vi "Parse Downlink.vi"(7 "CP_DATA IN":u8[](array[numeric]), 8 "error in (no error)":errorcluster, 9 "Parameters":string, 10 "EXID":u32 step=1 format="%06x", 11 "Command":T1) -> (0 "error out":errorcluster, 2 "Downlink":u8[][](array[numeric]) format="%02x")   [LabVIEW 2009]
uses:
  <vilib>/Utility/miscctls.llb/LVDateTimeRec.ctl
  Command List.ctl
  Typedef Command List.ctl
panel:
  in  "Command":T2 items=["Get xPG Status", "xPG Stimulation", "Select Program", "Increment Program Amplitude", "Decrement Program Amplitude", "Get PoP Constants", "Get PPC Constants", "Get Program Names", "Set Pulse Amplitude", "Increment Pulse Amplitude", "Decrement Pulse Amplitude", "Get Pulse Widths", "Set Pulse Widths", "Increment Pulse Width", "Decrement Pulse Width", "Get Program Frequency", "Set Program Frequency", "Increment Program Frequency", "Decrement Program Frequency", "reserved", "Charging Control", "Get xPG Identity", "Set xPG Identity", "Restore Program Defaults", "Get Program Definition", "Set Program Definition", "Get Program Constants", "Set Program Constants", "Get Configurable Device Parameters", "Set Configurable Device Parameters", "Get Pulse Constants", "Set Pulse Constants", "Get Lead Limits", "Set Lead Limits", "Get Channel Calibrations", "Set Channel Calibrations", "reserved", "reserved", "reserved", "reserved", "reserved", "reserved", "Get Stim Asic HV Calibrations", "Set Stim Asic HV Calibrations", "reserved", "reserved", "Get CP Data", "Set CP Data", "Clear Log", "Read Log", "Append Log", "Get Patient Program Runtime", "Set Patient Program Runtimec", "Impedance Measurement", "Enter Storage Mode", "Echo Short", "Echo Long", "Get General Calibration", "Set General Calibration", "Get Trim List", "Set Trim List", "Get Counter", "Set Counter", "Get Test Stimulation", "Set Test Stimulation", "Get Titration Stimulation", "Set Titration Stimulation", "Get Ramp Time", "Set Ramp Time", "Get VBAT", "Set Software Description Block", "Write Memory", "Read Memory", "Reset xPG", "Erase Flash Block", "Write Vectors", "Read Vectors", "Diagnostic Data", "Set Background Impedance", "Get Background Impedence ", "Undefined"]
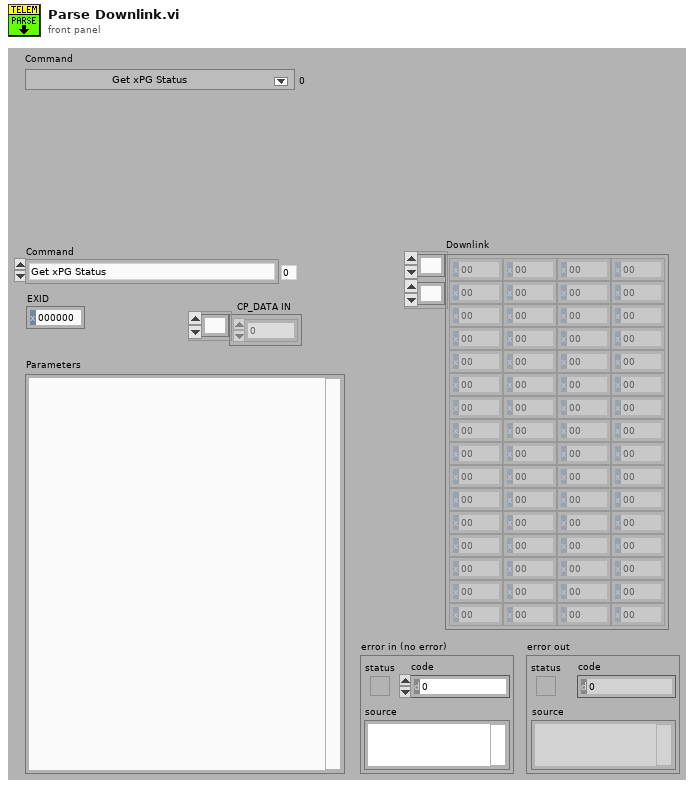
[diagram p1: front panel]
types:
  T1 = typedef "Typedef Command List.ctl" = enum16{"Get xPG Status", "xPG Stimulation", "Select Program", "Increment Program Amplitude", "Decrement Program Amplitude", "Get PoP Constants", "Get PPC Constants", "Get Program Names", "Set Pulse Amplitude", "Increment Pulse Amplitude", "Decrement Pulse Amplitude", "Get Pulse Widths", "Set Pulse Widths", "Increment Pulse Width", "Decrement Pulse Width", "Get Program Frequency", "Set Program Frequency", "Increment Program Frequency", "Decrement Program Frequency", "<reserved 1>", "Charging Control", "Get xPG Identity", "Set xPG Identity", "Restore Program Defaults", "Get Program Definition", "Set Program Definition", "Get Program Constants", "Set Program Constants", "Get Configurable Device Parameters", "Set Configurable Device Parameters", "Get Pulse Constants", "Set Pulse Constants", "Get Lead Limits", "Set Lead Limits", "Get Channel Calibrations", "Set Channel Calibrations", "<reserved 2>", "<reserved 3>", "<reserved 4>", "<reserved 5>", "<reserved 6>", "<reserved 7>", "Get Stim Asic HV Calibrations", "Set Stim Asic HV Calibrations", "<reserved 8>", "<reserved 9>", "Get CP Data", "Set CP Data", "Clear Log", "Read Log", "Append Log", "Get Patient Program Runtime", "Set Patient Program Runtime", "Impedance Measurement", "Enter Storage Mode", "Echo Short", "Echo Long", "Get General Calibration", "Set General Calibration", "Get Trim List", "Set Trim List", "Get Counter", "Set Counter", "Get Test Stimulation", "Set Test Stimulation", "Get Titration Stimulation", "Set Titration Stimulation", "Get Ramp Time", "Set Ramp Time", "Get VBAT", "Set Software Description Block", "Get Software Description Block", "Write Memory", "Read Memory", "Reset xPG", "Erase Flash Block", "Write Vectors", "Read Vectors", "Diagnostic Data", "Set Background Impedance", "Get Background Impedence ", "Undefined"}
  T2 = typedef "Command List.ctl" = u16
  T3 = enum16{"U8", "U16", "U32", "U64", "I8", "I16", "I32", "I64"}
  T4 = typedef "LVDateTimeRec.ctl" = cluster{"fractional second":dbl, "second":i32, "minute":i32, "hour":i32, "day of month":i32, "month":i32, "year":i32, "day of week":i32, "day of year":i32, "DST":i32}
  T5 = cluster{"CP_DATA IN[0]":u8, "CP_DATA IN[1]":u8, "CP_DATA IN[2]":u8, "CP_DATA IN[3]":u8, "CP_DATA IN[4]":u8, "CP_DATA IN[5]":u8, "CP_DATA IN[6]":u8, "CP_DATA IN[7]":u8, "CP_DATA IN[8]":u8, "CP_DATA IN[9]":u8, "CP_DATA IN[10]":u8, "CP_DATA IN[11]":u8, "CP_DATA IN[12]":u8, "CP_DATA IN[13]":u8, "CP_DATA IN[14]":u8, "CP_DATA IN[15]":u8, "CP_DATA IN[16]":u8, "CP_DATA IN[17]":u8, "CP_DATA IN[18]":u8, "CP_DATA IN[19]":u8, "CP_DATA IN[20]":u8, "CP_DATA IN[21]":u8, "CP_DATA IN[22]":u8, "CP_DATA IN[23]":u8, "CP_DATA IN[24]":u8, "CP_DATA IN[25]":u8, "CP_DATA IN[26]":u8, "CP_DATA IN[27]":u8, "CP_DATA IN[28]":u8, "CP_DATA IN[29]":u8, "CP_DATA IN[30]":u8, "CP_DATA IN[31]":u8, "CP_DATA IN[32]":u8, "CP_DATA IN[33]":u8, "CP_DATA IN[34]":u8, "CP_DATA IN[35]":u8, "CP_DATA IN[36]":u8, "CP_DATA IN[37]":u8, "CP_DATA IN[38]":u8, "CP_DATA IN[39]":u8, "CP_DATA IN[40]":u8, "CP_DATA IN[41]":u8, "CP_DATA IN[42]":u8, "CP_DATA IN[43]":u8, "CP_DATA IN[44]":u8, "CP_DATA IN[45]":u8, "CP_DATA IN[46]":u8, "CP_DATA IN[47]":u8, "CP_DATA IN[48]":u8, "CP_DATA IN[49]":u8, "CP_DATA IN[50]":u8, "CP_DATA IN[51]":u8, "CP_DATA IN[52]":u8, "CP_DATA IN[53]":u8, "CP_DATA IN[54]":u8, "CP_DATA IN[55]":u8, "CP_DATA IN[56]":u8, "CP_DATA IN[57]":u8, "CP_DATA IN[58]":u8, "CP_DATA IN[59]":u8, "CP_DATA IN[60]":u8, "CP_DATA IN[61]":u8, "CP_DATA IN[62]":u8, "CP_DATA IN[63]":u8, "CP_DATA IN[64]":u8, "CP_DATA IN[65]":u8, "CP_DATA IN[66]":u8, "CP_DATA IN[67]":u8, "CP_DATA IN[68]":u8, "CP_DATA IN[69]":u8, "CP_DATA IN[70]":u8, "CP_DATA IN[71]":u8, "CP_DATA IN[72]":u8, "CP_DATA IN[73]":u8, "CP_DATA IN[74]":u8, "CP_DATA IN[75]":u8, "CP_DATA IN[76]":u8, "CP_DATA IN[77]":u8, "CP_DATA IN[78]":u8, "CP_DATA IN[79]":u8, "CP_DATA IN[80]":u8, "CP_DATA IN[81]":u8, "CP_DATA IN[82]":u8, "CP_DATA IN[83]":u8, "CP_DATA IN[84]":u8, "CP_DATA IN[85]":u8, "CP_DATA IN[86]":u8, "CP_DATA IN[87]":u8, "CP_DATA IN[88]":u8, "CP_DATA IN[89]":u8, "CP_DATA IN[90]":u8, "CP_DATA IN[91]":u8, "CP_DATA IN[92]":u8, "CP_DATA IN[93]":u8, "CP_DATA IN[94]":u8, "CP_DATA IN[95]":u8, "CP_DATA IN[96]":u8, "CP_DATA IN[97]":u8, "CP_DATA IN[98]":u8, "CP_DATA IN[99]":u8, "CP_DATA IN[100]":u8, "CP_DATA IN[101]":u8, "CP_DATA IN[102]":u8, "CP_DATA IN[103]":u8, "CP_DATA IN[104]":u8, "CP_DATA IN[105]":u8, "CP_DATA IN[106]":u8, "CP_DATA IN[107]":u8, "CP_DATA IN[108]":u8, "CP_DATA IN[109]":u8, "CP_DATA IN[110]":u8, "CP_DATA IN[111]":u8, "CP_DATA IN[112]":u8, "CP_DATA IN[113]":u8, "CP_DATA IN[114]":u8, "CP_DATA IN[115]":u8, "CP_DATA IN[116]":u8, "CP_DATA IN[117]":u8, "CP_DATA IN[118]":u8, "CP_DATA IN[119]":u8, "CP_DATA IN[120]":u8, "CP_DATA IN[121]":u8, "CP_DATA IN[122]":u8, "CP_DATA IN[123]":u8, "CP_DATA IN[124]":u8, "CP_DATA IN[125]":u8, "CP_DATA IN[126]":u8, "CP_DATA IN[127]":u8, "CP_DATA IN[128]":u8, "CP_DATA IN[129]":u8, "CP_DATA IN[130]":u8, "CP_DATA IN[131]":u8, "CP_DATA IN[132]":u8, "CP_DATA IN[133]":u8, "CP_DATA IN[134]":u8, "CP_DATA IN[135]":u8, "CP_DATA IN[136]":u8, "CP_DATA IN[137]":u8, "CP_DATA IN[138]":u8, "CP_DATA IN[139]":u8, "CP_DATA IN[140]":u8, "CP_DATA IN[141]":u8, "CP_DATA IN[142]":u8, "CP_DATA IN[143]":u8, "CP_DATA IN[144]":u8, "CP_DATA IN[145]":u8, "CP_DATA IN[146]":u8, "CP_DATA IN[147]":u8, "CP_DATA IN[148]":u8, "CP_DATA IN[149]":u8, "CP_DATA IN[150]":u8, "CP_DATA IN[151]":u8, "CP_DATA IN[152]":u8, "CP_DATA IN[153]":u8, "CP_DATA IN[154]":u8, "CP_DATA IN[155]":u8, "CP_DATA IN[156]":u8, "CP_DATA IN[157]":u8, "CP_DATA IN[158]":u8, "CP_DATA IN[159]":u8, "CP_DATA IN[160]":u8, "CP_DATA IN[161]":u8, "CP_DATA IN[162]":u8, "CP_DATA IN[163]":u8, "CP_DATA IN[164]":u8, "CP_DATA IN[165]":u8, "CP_DATA IN[166]":u8, "CP_DATA IN[167]":u8, "CP_DATA IN[168]":u8, "CP_DATA IN[169]":u8, "CP_DATA IN[170]":u8, "CP_DATA IN[171]":u8, "CP_DATA IN[172]":u8, "CP_DATA IN[173]":u8, "CP_DATA IN[174]":u8, "CP_DATA IN[175]":u8, "CP_DATA IN[176]":u8, "CP_DATA IN[177]":u8, "CP_DATA IN[178]":u8, "CP_DATA IN[179]":u8, "CP_DATA IN[180]":u8, "CP_DATA IN[181]":u8, "CP_DATA IN[182]":u8, "CP_DATA IN[183]":u8, "CP_DATA IN[184]":u8, "CP_DATA IN[185]":u8, "CP_DATA IN[186]":u8, "CP_DATA IN[187]":u8, "CP_DATA IN[188]":u8, "CP_DATA IN[189]":u8, "CP_DATA IN[190]":u8, "CP_DATA IN[191]":u8, "CP_DATA IN[192]":u8, "CP_DATA IN[193]":u8, "CP_DATA IN[194]":u8, "CP_DATA IN[195]":u8, "CP_DATA IN[196]":u8, "CP_DATA IN[197]":u8, "CP_DATA IN[198]":u8, "CP_DATA IN[199]":u8, "CP_DATA IN[200]":u8, "CP_DATA IN[201]":u8, "CP_DATA IN[202]":u8, "CP_DATA IN[203]":u8, "CP_DATA IN[204]":u8, "CP_DATA IN[205]":u8, "CP_DATA IN[206]":u8, "CP_DATA IN[207]":u8, "CP_DATA IN[208]":u8, "CP_DATA IN[209]":u8, "CP_DATA IN[210]":u8, "CP_DATA IN[211]":u8, "CP_DATA IN[212]":u8, "CP_DATA IN[213]":u8, "CP_DATA IN[214]":u8, "CP_DATA IN[215]":u8, "CP_DATA IN[216]":u8, "CP_DATA IN[217]":u8, "CP_DATA IN[218]":u8, "CP_DATA IN[219]":u8, "CP_DATA IN[220]":u8, "CP_DATA IN[221]":u8, "CP_DATA IN[222]":u8, "CP_DATA IN[223]":u8, "CP_DATA IN[224]":u8, "CP_DATA IN[225]":u8, "CP_DATA IN[226]":u8, "CP_DATA IN[227]":u8, "CP_DATA IN[228]":u8, "CP_DATA IN[229]":u8, "CP_DATA IN[230]":u8, "CP_DATA IN[231]":u8, "CP_DATA IN[232]":u8, "CP_DATA IN[233]":u8, "CP_DATA IN[234]":u8, "CP_DATA IN[235]":u8, "CP_DATA IN[236]":u8, "CP_DATA IN[237]":u8, "CP_DATA IN[238]":u8, "CP_DATA IN[239]":u8, "CP_DATA IN[240]":u8, "CP_DATA IN[241]":u8, "CP_DATA IN[242]":u8, "CP_DATA IN[243]":u8, "CP_DATA IN[244]":u8, "CP_DATA IN[245]":u8, "CP_DATA IN[246]":u8, "CP_DATA IN[247]":u8, "CP_DATA IN[248]":u8, "CP_DATA IN[249]":u8, "CP_DATA IN[250]":u8, "CP_DATA IN[251]":u8, "CP_DATA IN[252]":u8, "CP_DATA IN[253]":u8, "CP_DATA IN[254]":u8, "CP_DATA IN[255]":u8}
  T6 = cluster{"DATA[0]":u8, "DATA[1]":u8, "DATA[2]":u8, "DATA[3]":u8, "DATA[4]":u8, "DATA[5]":u8, "DATA[6]":u8, "DATA[7]":u8, "DATA[8]":u8, "DATA[9]":u8, "DATA[10]":u8, "DATA[11]":u8, "DATA[12]":u8, "DATA[13]":u8, "DATA[14]":u8}
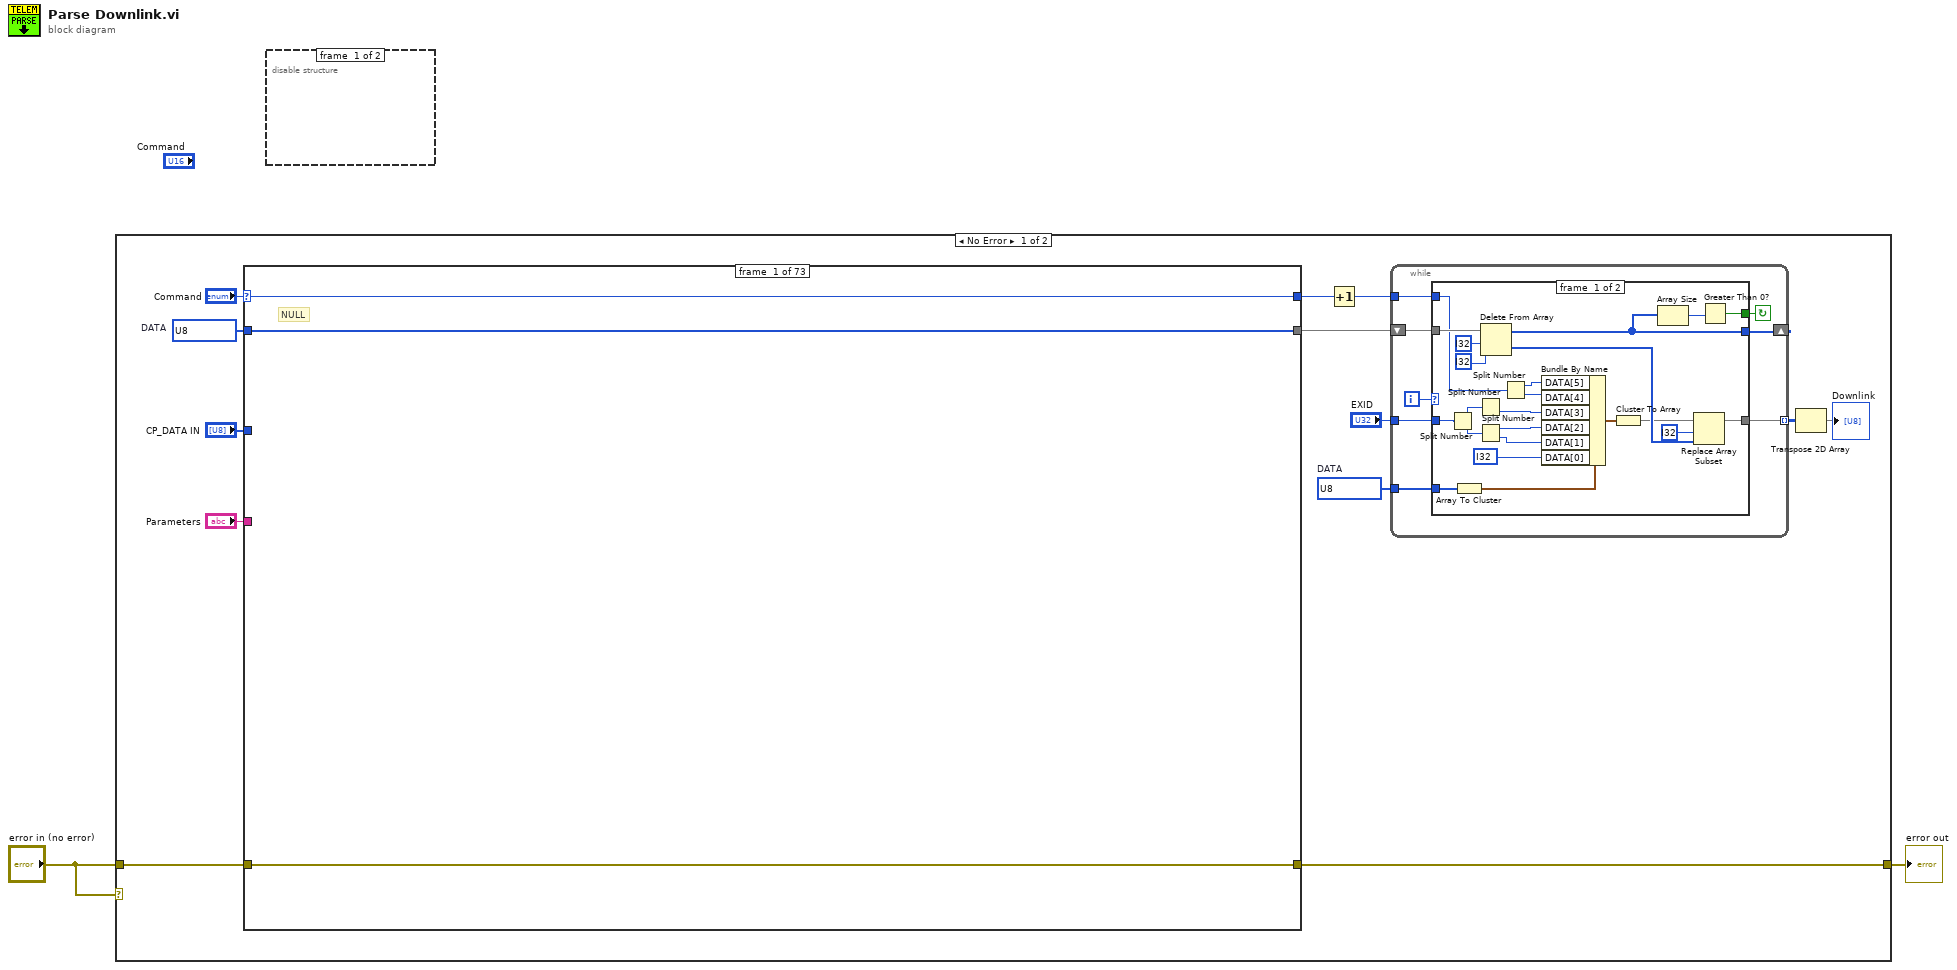
[diagram p0: block diagram]
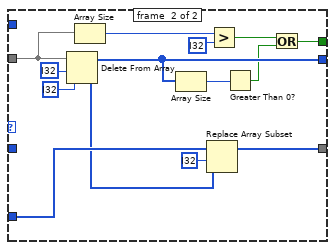
[diagram p3: hidden frame]
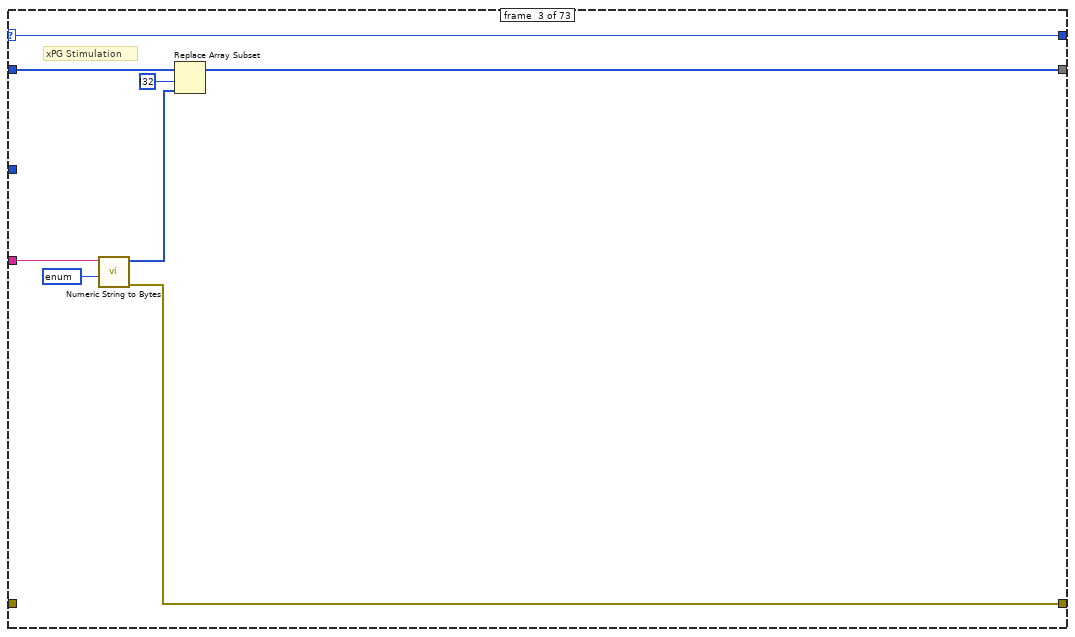
[diagram p5: hidden frame]
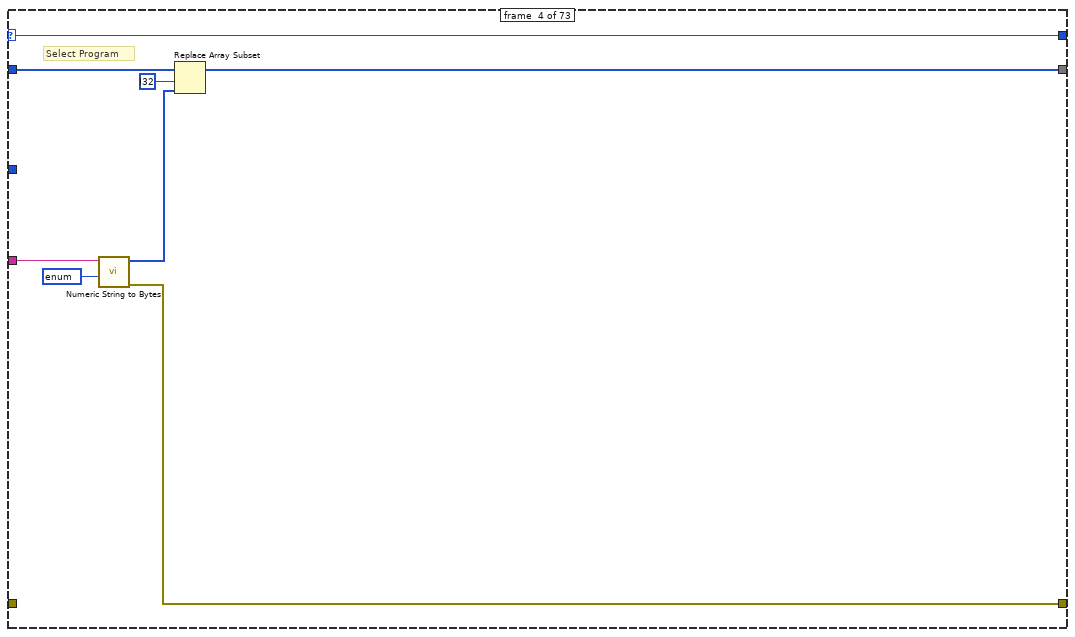
[diagram p6: hidden frame]
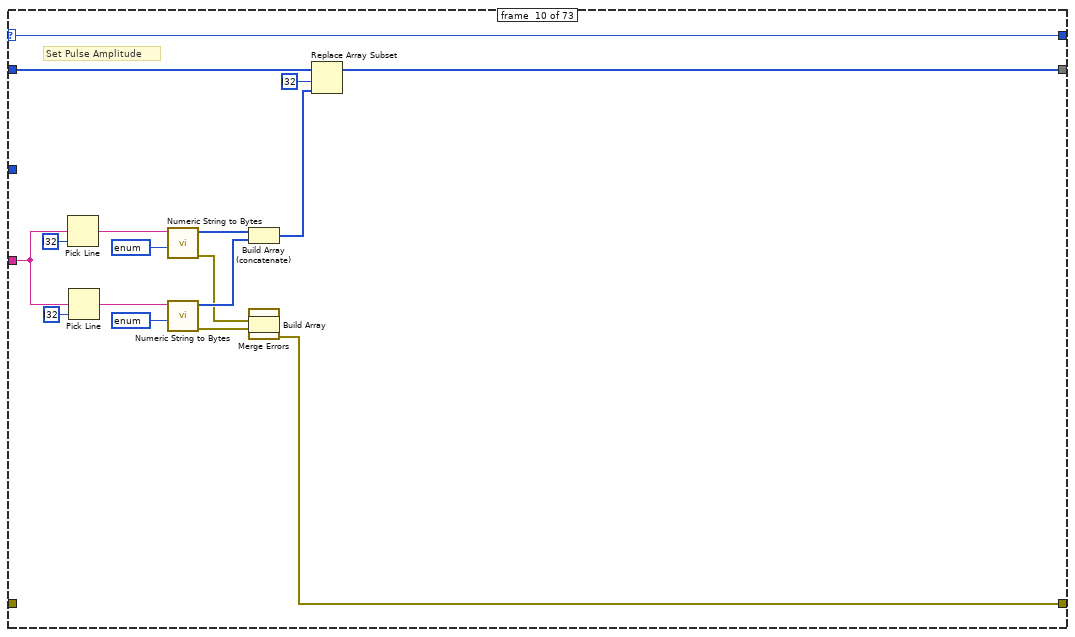
[diagram p12: hidden frame]
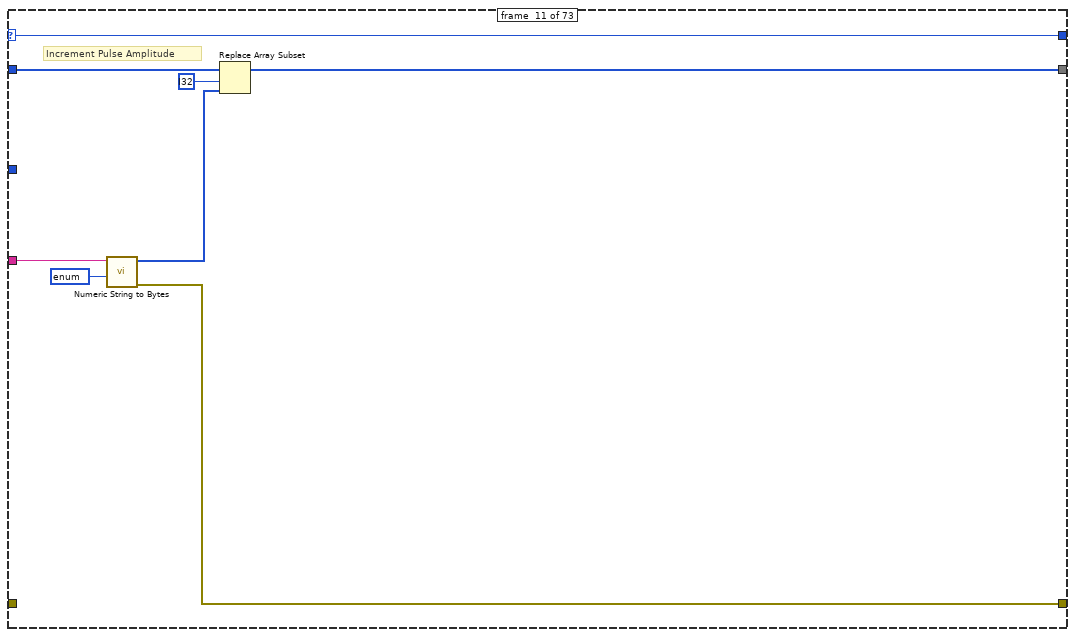
[diagram p13: hidden frame]
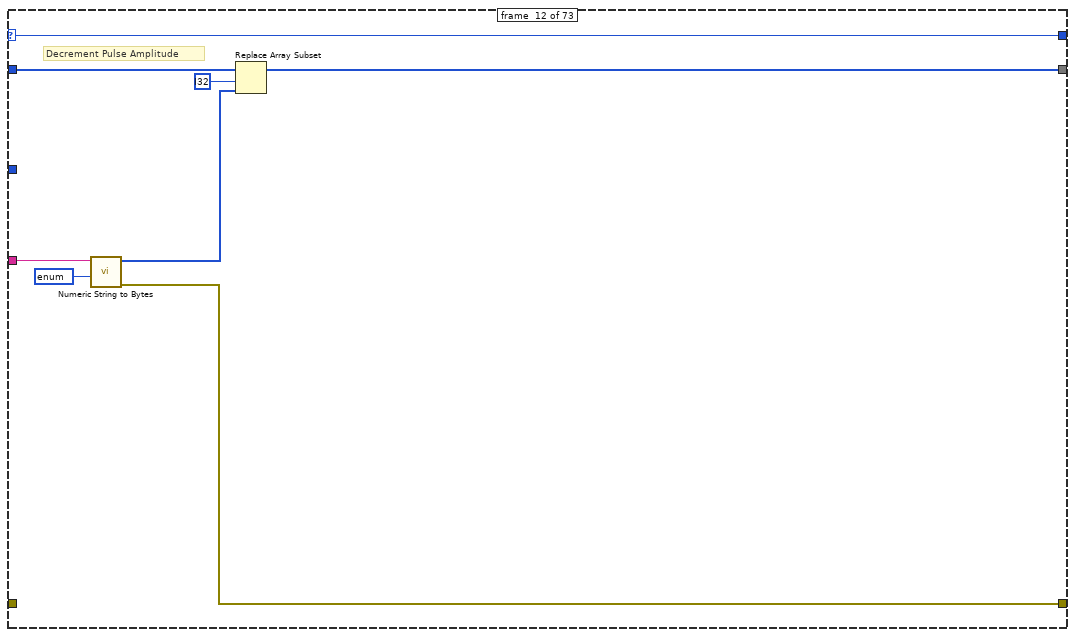
[diagram p14: hidden frame]
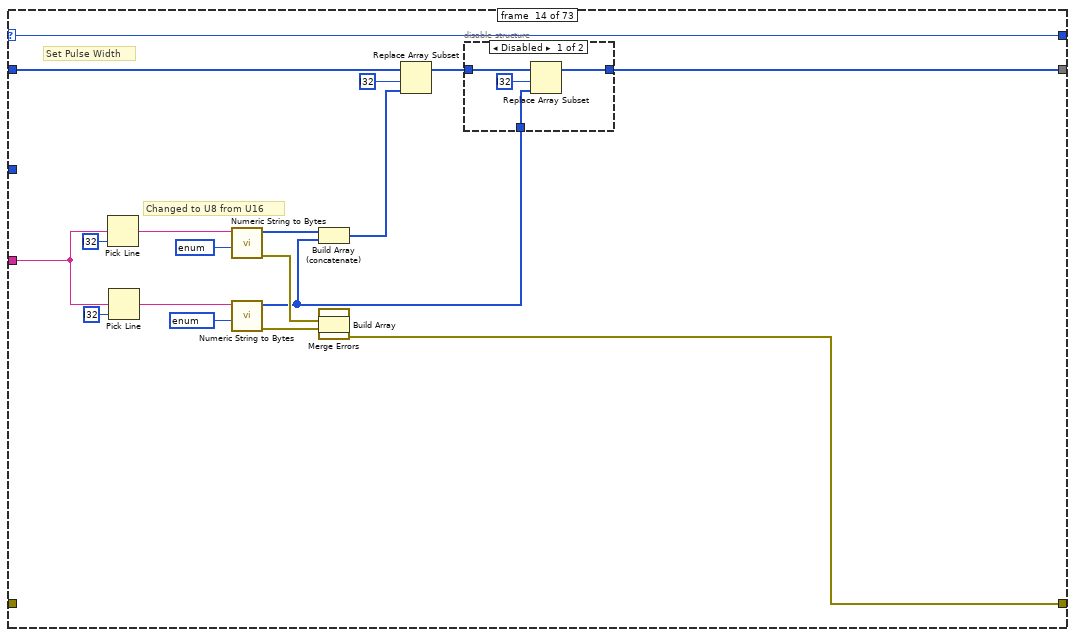
[diagram p16: hidden frame]
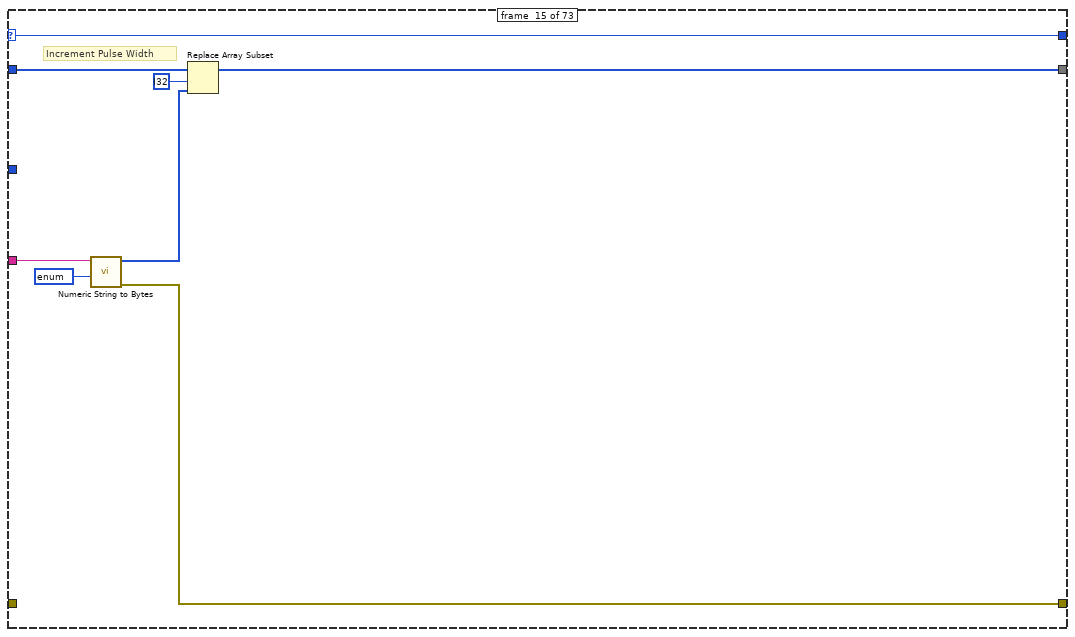
[diagram p18: hidden frame]
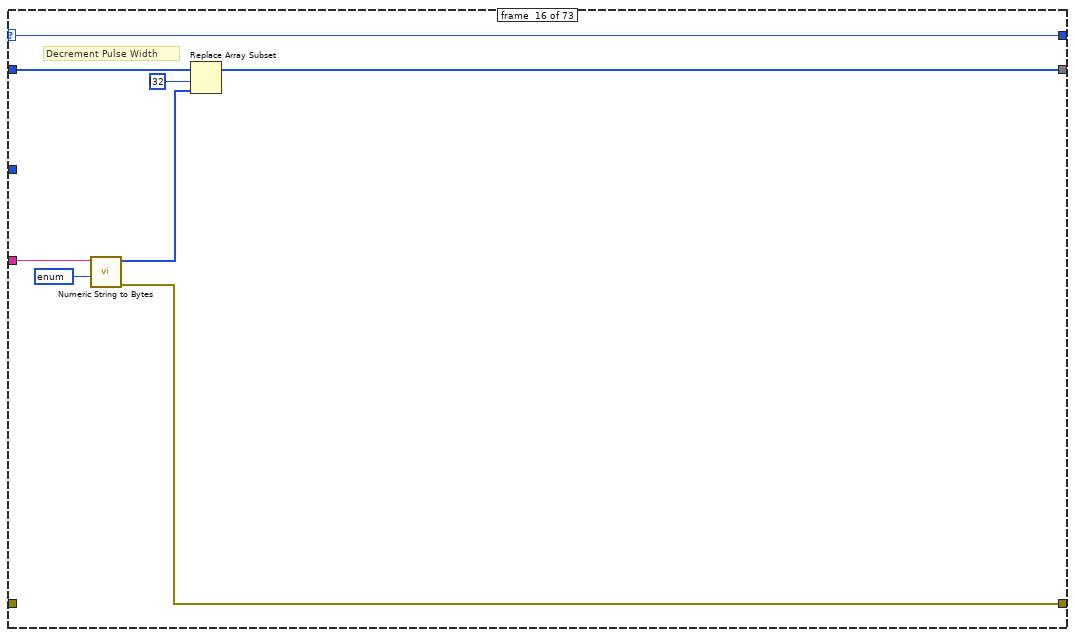
[diagram p19: hidden frame]
diagram:
  n1 = case shown="No Error" "error in (no error)" {
    tunnel: "error in (no error)" -> [w8 w1212]
    tunnel: [w7 w1212] -> w2
    frame #0 {
      w9 = u8[] ?  # DATA
      w10 = u8[] ?  # DATA
      n2 = case shown="\"Set Program Definition\"" "Command" {
        selector: "Command" -> [w63 w66 w74 w82 w85 w88 w91 w94 w97 w115 w123 w131 w134 w153 w166 w174 w177 w185 w188 w191 w194 w197 w224 w240 w248 w255 w395 w410 w423 w498 w516 w536 w547 w555 w566 w574 w585 w593 w609 w622 w630 w649 w688 w696 w715 w769 w772 w778 w784 w787 w794 w896 w918 w943 w962 w965 w989 w1046 w1066 w1099 w1107 w1110 w1113 w1116 w1135 w1153 w1156 w1159 w1162 w1165 w1183 w1208 w1211]
        tunnel: "Parameters" -> [_ _ w72 w80 _ _ _ _ _ w114 w121 w129 _ w141 w164 w172 _ w183 _ _ _ _ w222 w238 w246 w250 _ w398 _ w428 _ w523 _ w552 _ w571 _ w590 w607 w617 w628 w632 w653 w694 w698 w722 _ _ _ _ w790 w891 w906 w941 w945 _ w971 _ w1057 _ w1104 _ _ _ w1124 w1148 _ _ _ _ w1179 w1191 _]
        tunnel: [w63 w66 w74 w82 w85 w88 w91 w94 w97 w115 w123 w131 w134 w153 w166 w174 w177 w185 w188 w191 w194 w197 w224 w240 w248 w255 w395 w410 w423 w498 w516 w536 w547 w555 w566 w574 w585 w593 w609 w622 w630 w649 w688 w696 w715 w769 w772 w778 w784 w787 w794 w896 w918 w943 w962 w965 w989 w1046 w1066 w1099 w1107 w1110 w1113 w1116 w1135 w1153 w1156 w1159 w1162 w1165 w1183 w1208 w1211] -> w15
        tunnel: [w62 w65 w70 w78 w84 w87 w90 w93 w96 w107 w119 w127 w133 w139 w162 w170 w176 w181 w187 w190 w193 w196 w209 w236 w244 w251 w394 w408 w422 w495 w515 w533 w546 w550 w565 w569 w584 w588 w605 w616 w626 w647 w686 w692 w713 w767 w771 w774 w780 w786 w791 w889 w913 w939 w960 w963 w967 w1044 w1052 w1097 w1101 w1108 w1111 w1114 w1123 w1137 w1154 w1157 w1160 w1163 w1167 w1199 w1210] -> w13
        tunnel: w9 -> [w62 w65 w73 w81 w84 w87 w90 w93 w96 w106 w122 w130 w133 w146 w165 w173 w176 w184 w187 w190 w193 w196 w210 w239 w247 _ w394 _ w422 _ w515 _ w546 _ w565 _ w584 _ w608 _ w629 w648 w687 w695 w714 w768 w771 _ _ w786 _ w892 _ w942 w961 w963 _ w1044 _ w1097 w1103 w1108 w1111 w1114 _ w1138 w1154 w1157 w1160 w1163 w1170 _ w1210]
        tunnel: w8 -> [w61 w64 _ _ w83 w86 w89 w92 w95 _ _ _ w132 _ _ _ w175 _ w186 w189 w192 w195 _ _ _ w253 w393 _ w421 _ w514 _ w545 _ w564 _ w583 _ _ _ _ _ _ _ _ _ w770 w773 w779 w785 _ _ _ _ _ w964 _ w1045 _ w1098 _ w1109 w1112 w1115 _ _ w1155 w1158 w1161 w1164 _ _ w1209]
        tunnel: [w61 w64 w71 w79 w83 w86 w89 w92 w95 w99 w120 w128 w132 w142 w163 w171 w175 w182 w186 w189 w192 w195 w199 w237 w245 w252 w393 w401 w421 w496 w514 w532 w545 w553 w564 w572 w583 w591 w606 w621 w627 w633 w672 w693 w699 w753 w770 w773 w779 w785 w792 w890 w917 w940 w946 w964 w969 w1045 w1048 w1098 w1100 w1109 w1112 w1115 w1122 w1139 w1155 w1158 w1161 w1164 w1171 w1185 w1209] -> w7
        tunnel: "CP_DATA IN" -> [_ _ _ _ _ _ _ _ _ _ _ _ _ _ _ _ _ _ _ _ _ _ _ _ _ _ _ _ _ _ _ _ _ _ _ _ _ _ _ w613 _ _ _ _ _ _ _ w777 w783 _ _ _ _ _ _ _ _ _ _ _ _ _ _ _ w1119 _ _ _ _ _ _ _ _]
        frame #0 {
          # "NULL"
        }
        frame #1 {
          # "Get xPG Status"
        }
        frame #2 {
          # "xPG Stimulation"
          n3 = call "Numeric String to Bytes.vi"("Type"=T3 ?, "String"=w72) -> ("error out"=w71:errorcluster, "Byte Data"=w68:u8[])  [unwired: 8 in]
          n4 = Replace Array Subset(array=w73, new element=w68, index=i32 ?) -> (w70:u8[])
        }
        frame #3 {
          # "Select Program"
          n5 = call "Numeric String to Bytes.vi"("Type"=T3 ?, "String"=w80) -> ("error out"=w79:errorcluster, "Byte Data"=w76:u8[])  [unwired: 8 in]
          n6 = Replace Array Subset(array=w81, new element=w76, index=i32 ?) -> (w78:u8[])
        }
        frame #4 {
          # "Increment Program Amplitude"
        }
        frame #5 {
          # "Decrement Program Amplitude"
        }
        frame #6 {
          # "Get PoP Constants"
        }
        frame #7 {
          # "Get PPC Constants"
        }
        frame #8 {
          # "Get Program Names"
        }
        frame #9 {
          # "Set Pulse Amplitude"
          n7 = Pick Line(multi-line string=w114, line index=i32 ?) -> (output string=w108:string)  [unwired: 1 in]
          n8 = Pick Line(multi-line string=w114, line index=i32 ?) -> (output string=w109:string)  [unwired: 1 in]
          n9 = call "Numeric String to Bytes.vi"("Type"=T3 ?, "String"=w108) -> ("error out"=w101:errorcluster, "Byte Data"=w105:u8[])  [unwired: 8 in]
          n10 = call "Numeric String to Bytes.vi"("Type"=T3 ?, "String"=w109) -> ("error out"=w100:errorcluster, "Byte Data"=w104:u8[])  [unwired: 8 in]
          n11 = Build Array (concatenate)(w105, w104) -> (w102:u8[])
          n12 = Build Array(w101, w100) -> (w98:errorcluster[])
          n13 = call <vilib>:"Merge Errors.vi"("error array in"=w98) -> ("error out"=w99:errorcluster)  [unwired: 6 in]
          n14 = Replace Array Subset(array=w106, new element=w102, index=i32 ?) -> (w107:u8[])
        }
        frame #10 {
          # "Increment Pulse Amplitude"
          n15 = call "Numeric String to Bytes.vi"("Type"=T3 ?, "String"=w121) -> ("error out"=w120:errorcluster, "Byte Data"=w117:u8[])  [unwired: 8 in]
          n16 = Replace Array Subset(array=w122, new element=w117, index=i32 ?) -> (w119:u8[])
        }
        frame #11 {
          # "Decrement Pulse Amplitude"
          n17 = call "Numeric String to Bytes.vi"("Type"=T3 ?, "String"=w129) -> ("error out"=w128:errorcluster, "Byte Data"=w125:u8[])  [unwired: 8 in]
          n18 = Replace Array Subset(array=w130, new element=w125, index=i32 ?) -> (w127:u8[])
        }
        frame #12 {
          # "Get Pulse Widths"
        }
        frame #13 {
          # "Changed to U8 from U16"
          # "Set Pulse Width"
          n19 = Pick Line(multi-line string=w141, line index=i32 ?) -> (output string=w147:string)  [unwired: 1 in]
          n20 = Pick Line(multi-line string=w141, line index=i32 ?) -> (output string=w148:string)  [unwired: 1 in]
          n21 = call "Numeric String to Bytes.vi"("Type"=T3 ?, "String"=w147) -> ("error out"=w144:errorcluster, "Byte Data"=w138:u8[])  [unwired: 8 in]
          n22 = call "Numeric String to Bytes.vi"("Type"=T3 ?, "String"=w148) -> ("error out"=w143:errorcluster, "Byte Data"=w137:u8[])  [unwired: 8 in]
          n23 = Build Array (concatenate)(w138, w137) -> (w136:u8[])
          n24 = Build Array(w144, w143) -> (w135:errorcluster[])
          n25 = call <vilib>:"Merge Errors.vi"("error array in"=w135) -> ("error out"=w142:errorcluster)  [unwired: 6 in]
          n26 = Replace Array Subset(array=w146, new element=w136, index=i32 ?) -> (w140:u8[])
          n27 = disable-structure shown="Disabled" {
            disable-tunnel: w137 -> [w156 _]
            disable-tunnel: w140 -> [w155 w158]
            disable-tunnel: [w154 w158] -> w139
            frame #0 {
              n28 = Replace Array Subset(array=w155, new element=w156, index=i32 ?) -> (w154:u8[])
            }
            frame #1 {
            }
          }
        }
        frame #14 {
          # "Increment Pulse Width"
          n29 = call "Numeric String to Bytes.vi"("Type"=T3 ?, "String"=w164) -> ("error out"=w163:errorcluster, "Byte Data"=w160:u8[])  [unwired: 8 in]
          n30 = Replace Array Subset(array=w165, new element=w160, index=i32 ?) -> (w162:u8[])
        }
        frame #15 {
          # "Decrement Pulse Width"
          n31 = call "Numeric String to Bytes.vi"("Type"=T3 ?, "String"=w172) -> ("error out"=w171:errorcluster, "Byte Data"=w168:u8[])  [unwired: 8 in]
          n32 = Replace Array Subset(array=w173, new element=w168, index=i32 ?) -> (w170:u8[])
        }
        frame #16 {
          # "Get Program Frequency"
        }
        frame #17 {
          # "Set Program Frequency"
          n33 = call "Numeric String to Bytes.vi"("Type"=T3 ?, "String"=w183) -> ("error out"=w182:errorcluster, "Byte Data"=w179:u8[])  [unwired: 8 in]
          n34 = Replace Array Subset(array=w184, new element=w179, index=i32 ?) -> (w181:u8[])
        }
        frame #18 {
          # "Increment Program Frequency"
        }
        frame #19 {
          # "Decrement Program Frequency"
        }
        frame #20 {
          # "Charging Control"
        }
        frame #21 {
          # "Get xPG Identity"
        }
        frame #22 {
          w216 = u8[] ?  # DATA
          w217 = u8[] ?  # DATA
          # "Set xPG Identity"
          n35 = Pick Line(multi-line string=w222, line index=i32 ?) -> (output string=w205:string)  [unwired: 1 in]
          n36 = Pick Line(multi-line string=w222, line index=i32 ?) -> (output string=w202:string)  [unwired: 1 in]
          n37 = for {
            N: i32 ? -> [_]
            tunnel: w222 -> [w231]
            shift-right: [w227] -> w213
            shift-left: w210 -> [w228]
            tunnel: [w225] -> w200 mode=indexing
            i -> [w232]
            n38 = Pick Line(multi-line string=w231, line index=w232) -> (output string=w230:string)  [unwired: 1 in]
            n39 = call "Numeric String to Bytes.vi"("Type"=T3 ?, "String"=w230) -> ("error out"=w225:errorcluster, "Byte Data"=w226:u8[])  [unwired: 8 in]
            n40 = Build Array (concatenate)(w228, w226) -> (w227:u8[])
          }
          n41 = Match Pattern(string=w205, regular expression=string ?) -> (after substring=w204:string)  [unwired: 1 in, 3 out]
          n42 = Match Pattern(string=w202, regular expression=string ?) -> (after substring=w201:string)  [unwired: 1 in, 3 out]
          n43 = call <vilib>:"Trim Whitespace.vi"("string"=w204) -> ("trimmed string"=w219:string)  [unwired: 1 in]
          n44 = call <vilib>:"Trim Whitespace.vi"("string"=w201) -> ("trimmed string"=w218:string)  [unwired: 1 in]
          n45 = String To Byte Array(string=w219) -> (unsigned byte array=w214:u8[])
          n46 = String To Byte Array(string=w218) -> (unsigned byte array=w215:u8[])
          n47 = Replace Array Subset(array=w217, new element=w214, index=i32 ?) -> (w212:u8[])
          n48 = Replace Array Subset(array=w216, new element=w215, index=i32 ?) -> (w211:u8[])
          n49 = Build Array (concatenate)(w213, w212, w211) -> (w209:u8[])
          n50 = Build Array (concatenate)(w200) -> (w198:errorcluster[])
          n51 = call <vilib>:"Merge Errors.vi"("error array in"=w198) -> ("error out"=w199:errorcluster)  [unwired: 6 in]
        }
        frame #23 {
          # "Restore Program Defaults"
          n52 = call "Numeric String to Bytes.vi"("Type"=T3 ?, "String"=w238) -> ("error out"=w237:errorcluster, "Byte Data"=w234:u8[])  [unwired: 8 in]
          n53 = Replace Array Subset(array=w239, new element=w234, index=i32 ?) -> (w236:u8[])
        }
        frame #24 {
          # "Get Program Definition"
          n54 = call "Numeric String to Bytes.vi"("Type"=T3 ?, "String"=w246) -> ("error out"=w245:errorcluster, "Byte Data"=w242:u8[])  [unwired: 8 in]
          n55 = Replace Array Subset(array=w247, new element=w242, index=i32 ?) -> (w244:u8[])
        }
        frame #25 {
          w254 = u8[] ?  # DATA
          # "Set Program Definition"
          n56 = while {
            shift-right: [w259] -> w251
            shift-left: w254 -> [w260]
            shift-right: [w265] -> w252
            shift-left: w253 -> [w266]
            tunnel: w250 -> [w258]
            shift-right: [w256] -> _
            shift-left: i32 ? -> [w257]
            i -> [w261]
            stop <- w262 stop-if-true
            n57 = case shown="0" w261 {
              tunnel: w266 -> [w274 w328]
              tunnel: [w273 w327] -> w265
              tunnel: [bool ? ("status") bool ? ("status")] -> w263
              tunnel: w260 -> [w289 w331]
              tunnel: [w288 w330] -> w259
              tunnel: w258 -> [w291 w325]
              tunnel: w257 -> [_ w326]
              tunnel: [i32 ? ("line index") w323] -> w256
              frame #0 {
                w305 = u8[] ?  # DATA
                # "Changed to U8 from U16"
                n58 = Pick Line(multi-line string=w291, line index=i32 ?) -> (output string=w298:string)  [unwired: 1 in]
                n59 = Pick Line(multi-line string=w291, line index=i32 ?) -> (output string=w299:string)  [unwired: 1 in]
                n60 = Pick Line(multi-line string=w291, line index=i32 ?) -> (output string=w300:string)  [unwired: 1 in]
                n61 = Pick Line(multi-line string=w291, line index=i32 ?) -> (output string=w270:string)  [unwired: 1 in]
                n62 = Pick Line(multi-line string=w291, line index=i32 ?) -> (output string=w295:string)  [unwired: 1 in]
                n63 = Pick Line(multi-line string=w291, line index=i32 ?) -> (output string=w292:string)  [unwired: 1 in]
                n64 = for {
                  N: i32 ? -> [_]
                  tunnel: w291 -> [w322]
                  shift-right: [w314] -> w283
                  shift-left: w289 -> [w315]
                  tunnel: [w313] -> w268 mode=indexing
                  i -> [w320]
                  n65 = Add(x=i32 ? ("line index"), y=w320) -> (x+y=w319:i32)
                  n66 = Pick Line(multi-line string=w322, line index=w319) -> (output string=w317:string)  [unwired: 1 in]
                  n67 = call "Numeric String to Bytes.vi"("Type"=T3 ?, "String"=w317) -> ("error out"=w313:errorcluster, "Byte Data"=w316:u8[])  [unwired: 8 in]
                  n68 = Build Array (concatenate)(w315, w316) -> (w314:u8[])
                }
                n69 = Match Pattern(string=w270, regular expression=string ?) -> (after substring=w269:string)  [unwired: 1 in, 3 out]
                n70 = call <vilib>:"Trim Whitespace.vi"("string"=w269) -> ("trimmed string"=w308:string)  [unwired: 1 in]
                n71 = call "Numeric String to Bytes.vi"("Type"=T3 ?, "String"=w298) -> ("error out"=w279:errorcluster, "Byte Data"=w287:u8[])  [unwired: 8 in]
                n72 = call "Numeric String to Bytes.vi"("Type"=T3 ?, "String"=w299) -> ("error out"=w278:errorcluster, "Byte Data"=w286:u8[])  [unwired: 8 in]
                n73 = call "Numeric String to Bytes.vi"("Type"=T3 ?, "String"=w300) -> ("error out"=w277:errorcluster, "Byte Data"=w285:u8[])  [unwired: 8 in]
                n74 = call "Numeric String to Bytes.vi"("Type"=T3 ?, "String"=w295) -> ("error out"=w276:errorcluster, "Byte Data"=w282:u8[])  [unwired: 8 in]
                n75 = call "Numeric String to Bytes.vi"("Type"=T3 ?, "String"=w292) -> ("error out"=w275:errorcluster, "Byte Data"=w281:u8[])  [unwired: 8 in]
                n76 = String To Byte Array(string=w308) -> (unsigned byte array=w307:u8[])
                n77 = Replace Array Subset(array=w305, new element=w307, index=i32 ?) -> (w284:u8[])
                n78 = Build Array (concatenate)(w289, w287, w286, w285, w284, w283, w282, w281) -> (w288:u8[])
                n79 = Build Array (concatenate)(w279, w278, w277, w268, w276, w275, w274) -> (w272:errorcluster[])
                n80 = Build Array (concatenate)(w272) -> (w267:errorcluster[])
                n81 = call <vilib>:"Merge Errors.vi"("error array in"=w267) -> ("error out"=w273:errorcluster)  [unwired: 6 in]
              }
              frame #1 {
                n82 = for {
                  N: i32 ? -> [_]
                  shift-right: [w348] -> w330
                  shift-left: w331 -> [w365]
                  shift-right: [w350] -> w327
                  shift-left: w328 -> [w357]
                  tunnel: w325 -> [w341]
                  shift-right: [w335] -> w323
                  shift-left: w326 -> [w342]
                  w340 = u8[] ?  # DATA
                  w333 = u8[] ?  # DATA
                  n83 = Increment(x=w342) -> (x+1=w336:i32)
                  n84 = Increment(x=w336) -> (x+1=w368:i32)
                  n85 = Pick Line(multi-line string=w341, line index=w342) -> (output string=w339:string)  [unwired: 1 in]
                  n86 = Pick Line(multi-line string=w341, line index=w336) -> (output string=w380:string)  [unwired: 1 in]
                  n87 = Increment(x=w368) -> (x+1=w369:i32)
                  n88 = Pick Line(multi-line string=w341, line index=w368) -> (output string=w381:string)  [unwired: 1 in]
                  n89 = Match Pattern(string=w339, regular expression=string ?) -> (after substring=w338:string)  [unwired: 1 in, 3 out]
                  n90 = Increment(x=w369) -> (x+1=w370:i32)
                  n91 = Pick Line(multi-line string=w341, line index=w369) -> (output string=w374:string)  [unwired: 1 in]
                  n92 = Increment(x=w370) -> (x+1=w371:i32)
                  n93 = Pick Line(multi-line string=w341, line index=w370) -> (output string=w375:string)  [unwired: 1 in]
                  n94 = call <vilib>:"Trim Whitespace.vi"("string"=w338) -> ("trimmed string"=w346:string)  [unwired: 1 in]
                  n95 = Increment(x=w371) -> (x+1=w367:i32)
                  n96 = Pick Line(multi-line string=w341, line index=w371) -> (output string=w376:string)  [unwired: 1 in]
                  n97 = Increment(x=w367) -> (x+1=w366:i32)
                  n98 = String To Byte Array(string=w346) -> (unsigned byte array=w345:u8[])
                  n99 = Pick Line(multi-line string=w341, line index=w367) -> (output string=w372:string)  [unwired: 1 in]
                  n100 = for {
                    N: i32 ? -> [_]
                    tunnel: w341 -> [w392]
                    shift-right: [w387] -> w358
                    shift-left: w340 -> [w388]
                    shift-right: [w385] -> w335
                    shift-left: w366 -> [w386]
                    tunnel: [w384] -> w334 mode=indexing
                    n101 = Pick Line(multi-line string=w392, line index=w386) -> (output string=w390:string)  [unwired: 1 in]
                    n102 = Increment(x=w386) -> (x+1=w385:i32)
                    n103 = call "Numeric String to Bytes.vi"("Type"=T3 ?, "String"=w390) -> ("error out"=w384:errorcluster, "Byte Data"=w389:u8[])  [unwired: 8 in]
                    n104 = Build Array (concatenate)(w388, w389) -> (w387:u8[])
                  }
                  n105 = Replace Array Subset(array=w333, new element=w345, index=i32 ?) -> (w343:u8[])
                  n106 = call "Numeric String to Bytes.vi"("Type"=T3 ?, "String"=w380) -> ("error out"=w356:errorcluster, "Byte Data"=w364:u8[])  [unwired: 8 in]
                  n107 = call "Numeric String to Bytes.vi"("Type"=T3 ?, "String"=w381) -> ("error out"=w355:errorcluster, "Byte Data"=w363:u8[])  [unwired: 8 in]
                  n108 = call "Numeric String to Bytes.vi"("Type"=T3 ?, "String"=w374) -> ("error out"=w354:errorcluster, "Byte Data"=w362:u8[])  [unwired: 8 in]
                  n109 = call "Numeric String to Bytes.vi"("Type"=T3 ?, "String"=w375) -> ("error out"=w353:errorcluster, "Byte Data"=w361:u8[])  [unwired: 8 in]
                  n110 = call "Numeric String to Bytes.vi"("Type"=T3 ?, "String"=w376) -> ("error out"=w352:errorcluster, "Byte Data"=w360:u8[])  [unwired: 8 in]
                  n111 = call "Numeric String to Bytes.vi"("Type"=T3 ?, "String"=w372) -> ("error out"=w351:errorcluster, "Byte Data"=w359:u8[])  [unwired: 8 in]
                  n112 = Build Array (concatenate)(w365, w343, w364, w363, w362, w361, w360, w359, w358) -> (w348:u8[])
                  n113 = Build Array (concatenate)(w357, w356, w355, w354, w353, w352, w351, w334) -> (w349:errorcluster[])
                  n114 = Build Array (concatenate)(w349) -> (w332:errorcluster[])
                  n115 = call <vilib>:"Merge Errors.vi"("error array in"=w332) -> ("error out"=w350:errorcluster)  [unwired: 6 in]
                }
              }
            }
            n116 = Unbundle By Name(w265) -> ("status"=w264:bool)
            n117 = Or(x=w263, y=w264) -> (x .or. y?=w262:bool)
          }
        }
        frame #26 {
          # "Get Program Constants"
        }
        frame #27 {
          w407 = u8[] ?  # DATA
          # "Set Program Constants"
          n118 = Pick Line(multi-line string=w398, line index=i32 ?) -> (output string=w404:string)  [unwired: 1 in]
          n119 = for {
            N: i32 ? -> [_]
            tunnel: w398 -> [w420]
            shift-right: [w413] -> w406
            shift-left: w407 -> [w414]
            tunnel: i32 ? -> [w415]
            tunnel: [w411] -> w400 mode=indexing
            i -> [w417]
            n120 = Add(x=w415, y=w417) -> (x+y=w416:i32)
            n121 = Pick Line(multi-line string=w420, line index=w416) -> (output string=w419:string)  [unwired: 1 in]
            n122 = call "Numeric String to Bytes.vi"("Type"=T3 ?, "String"=w419) -> ("error out"=w411:errorcluster, "Byte Data"=w412:u8[])  [unwired: 8 in]
            n123 = Build Array (concatenate)(w414, w412) -> (w413:u8[])
          }
          n124 = call "Numeric String to Bytes.vi"("Type"=T3 ?, "String"=w404) -> ("error out"=w399:errorcluster, "Byte Data"=w402:u8[])  [unwired: 8 in]
          n125 = Build Array (concatenate)(w402, w406) -> (w408:u8[])
          n126 = Build Array (concatenate)(w399, w400) -> (w396:errorcluster[])
          n127 = call <vilib>:"Merge Errors.vi"("error array in"=w396) -> ("error out"=w401:errorcluster)  [unwired: 6 in]
        }
        frame #28 {
          # "Get Configurable Device Parameters"
        }
        frame #29 {
          w446 = i32 ?
          w490 = u8[] ?  # DATA
          w497 = u8[] ?  # DATA
          # "Changed to U8 from U16"
          # "Set Configurable Device Parameters"
          n128 = Pick Line(multi-line string=w428, line index=i32 ?) -> (output string=w426:string)  [unwired: 1 in]
          n129 = Match Pattern(string=w426, regular expression=string ?) -> (after substring=w425:string)  [unwired: 1 in, 3 out]
          n130 = Scan From String(format string=string ?, input string=w425) -> (error out=w444:errorcluster, output 1=w454:i32, output 2=w453:i32, output 3=w452:i32, output 4=w451:i32, output 5=w450:i32, output 6=w449:i32, output 7=w455:string)  [unwired: 9 in, 2 out]
          n131 = case shown="\"PM\"" w455 {
            tunnel: w451 -> [w499 w501 w504]
            tunnel: [w499 w500 w503] -> w448
            frame #0 {
            }
            frame #1 {
              n132 = Subtract(x=w501, y=i32 ?) -> (x-y=w500:i32)
            }
            frame #2 {
              n133 = Add(x=w504, y=i32 ?) -> (x+y=w503:i32)
            }
          }
          n134 = for {
            N: i32 ? -> [_]
            tunnel: [w511] -> w489 mode=indexing
            tunnel: w428 -> [w510]
            shift-right: [w508] -> w484
            shift-left: w497 -> [w507]
            i -> [w509]
            n135 = Pick Line(multi-line string=w510, line index=w509) -> (output string=w512:string)  [unwired: 1 in]
            n136 = call "Numeric String to Bytes.vi"("Type"=T3 ?, "String"=w512) -> ("error out"=w511:errorcluster, "Byte Data"=w506:u8[])  [unwired: 8 in]
            n137 = Build Array (concatenate)(w507, w506) -> (w508:u8[])
          }
          n138 = Pick Line(multi-line string=w428, line index=i32 ?) -> (output string=w486:string)  [unwired: 1 in]
          n139 = Pick Line(multi-line string=w428, line index=i32 ?) -> (output string=w480:string)  [unwired: 1 in]
          n140 = Pick Line(multi-line string=w428, line index=i32 ?) -> (output string=w475:string)  [unwired: 1 in]
          n141 = Pick Line(multi-line string=w428, line index=i32 ?) -> (output string=w472:string)  [unwired: 1 in]
          n142 = Pick Line(multi-line string=w428, line index=i32 ?) -> (output string=w469:string)  [unwired: 1 in]
          n143 = Pick Line(multi-line string=w428, line index=i32 ?) -> (output string=w458:string)  [unwired: 1 in]
          n144 = Bundle By Name(cluster=T4 ? ("date time rec"), "month"=w454, "day of month"=w453, "year"=w452, "hour"=w448, "minute"=w450, "second"=w449, "day of week"=w446, "day of year"=w446, "DST"=w446, "fractional second"=w446) -> (w445:T4)
          n145 = Match Pattern(string=w486, regular expression=string ?) -> (after substring=w485:string)  [unwired: 1 in, 3 out]
          n146 = call "Numeric String to Bytes.vi"("Type"=T3 ?, "String"=w480) -> ("error out"=w478:errorcluster, "Byte Data"=w479:u8[])  [unwired: 8 in]
          n147 = call "Numeric String to Bytes.vi"("Type"=T3 ?, "String"=w475) -> ("error out"=w467:errorcluster, "Byte Data"=w464:u8[])  [unwired: 8 in]
          n148 = call "Numeric String to Bytes.vi"("Type"=T3 ?, "String"=w472) -> ("error out"=w466:errorcluster, "Byte Data"=w463:u8[])  [unwired: 8 in]
          n149 = call "Numeric String to Bytes.vi"("Type"=T3 ?, "String"=w469) -> ("error out"=w465:errorcluster, "Byte Data"=w462:u8[])  [unwired: 8 in]
          n150 = call "Numeric String to Bytes.vi"("Type"=T3 ?, "String"=w458) -> ("error out"=w432:errorcluster, "Byte Data"=w459:u8[])  [unwired: 8 in]
          n151 = call <vilib>:"Trim Whitespace.vi"("string"=w485) -> ("trimmed string"=w493:string)  [unwired: 1 in]
          n152 = String To Byte Array(string=w493) -> (unsigned byte array=w492:u8[])
          n153 = Date/Time To Seconds(2:w445) -> (0:w441:timestamp)  [unwired: 1 in]
          n154 = Replace Array Subset(array=w490, new element=w492, index=i32 ?) -> (w482:u8[])
          n155 = To Unsigned Quad Integer(1:w441) -> (0:w440:u64)
          n156 = Multiply(x=u64 ? ("y"), y=u64 ?) -> (x*y=w439:u64)
          n157 = Add(x=w440, y=w439) -> (x+y=w438:u64)
          n158 = Multiply(x=u64 ? ("y"), y=w438) -> (x*y=w436:u64)
          n159 = Number To Decimal String(number=w436) -> (decimal integer string=w433:string)  [unwired: 1 in]
          n160 = Concatenate Strings(string ? ("string"), w433) -> (w434:string)
          n161 = call "Numeric String to Bytes.vi"("Type"=T3 ?, "String"=w434) -> ("error out"=w431:errorcluster, "Byte Data"=w429:u8[])  [unwired: 8 in]
          n162 = Build Array (concatenate)(w484, w482, w479, w464, w463, w462, w429, w459) -> (w495:u8[])
          n163 = Build Array (concatenate)(w489, w478, w467, w466, w465, w444, w431, w432) -> (w488:errorcluster[])
          n164 = Build Array (concatenate)(w488) -> (w424:errorcluster[])
          n165 = call <vilib>:"Merge Errors.vi"("error array in"=w424) -> ("error out"=w496:errorcluster)  [unwired: 6 in]
        }
        frame #30 {
          # "Get Pulse Constants"
        }
        frame #31 {
          w518 = u8[] ?  # DATA
          # "Set Pulse Constants"
          n166 = for {
            N: i32 ? -> [_]
            tunnel: w523 -> [w543]
            shift-right: [w539] -> w534
            shift-left: w518 -> [w540]
            tunnel: [w537] -> w521 mode=indexing
            i -> [w544]
            n167 = Pick Line(multi-line string=w543, line index=w544) -> (output string=w542:string)  [unwired: 1 in]
            n168 = call "Numeric String to Bytes.vi"("Type"=T3 ?, "String"=w542) -> ("error out"=w537:errorcluster, "Byte Data"=w538:u8[])  [unwired: 8 in]
            n169 = Build Array (concatenate)(w540, w538) -> (w539:u8[])
          }
          n170 = Pick Line(multi-line string=w523, line index=i32 ?) -> (output string=w531:string)  [unwired: 1 in]
          n171 = Pick Line(multi-line string=w523, line index=i32 ?) -> (output string=w528:string)  [unwired: 1 in]
          n172 = call "Numeric String to Bytes.vi"("Type"=T3 ?, "String"=w531) -> ("error out"=w519:errorcluster, "Byte Data"=w524:u8[])  [unwired: 8 in]
          n173 = call "Numeric String to Bytes.vi"("Type"=T3 ?, "String"=w528) -> ("error out"=w522:errorcluster, "Byte Data"=w525:u8[])  [unwired: 8 in]
          n174 = Build Array (concatenate)(w534, w524, w525) -> (w533:u8[])
          n175 = Build Array (concatenate)(w521, w519, w522) -> (w520:errorcluster[])
          n176 = Build Array (concatenate)(w520) -> (w517:errorcluster[])
          n177 = call <vilib>:"Merge Errors.vi"("error array in"=w517) -> ("error out"=w532:errorcluster)  [unwired: 6 in]
        }
        frame #32 {
          # "Get Lead Limits"
        }
        frame #33 {
          w549 = u8[] ?  # DATA
          # "Set Lead Limits"
          n178 = for {
            N: i32 ? -> [_]
            tunnel: w552 -> [w562]
            shift-right: [w558] -> w550
            shift-left: w549 -> [w559]
            tunnel: [w556] -> w551 mode=indexing
            i -> [w563]
            n179 = Pick Line(multi-line string=w562, line index=w563) -> (output string=w561:string)  [unwired: 1 in]
            n180 = call "Numeric String to Bytes.vi"("Type"=T3 ?, "String"=w561) -> ("error out"=w556:errorcluster, "Byte Data"=w557:u8[])  [unwired: 8 in]
            n181 = Build Array (concatenate)(w559, w557) -> (w558:u8[])
          }
          n182 = Build Array (concatenate)(w551) -> (w548:errorcluster[])
          n183 = call <vilib>:"Merge Errors.vi"("error array in"=w548) -> ("error out"=w553:errorcluster)  [unwired: 6 in]
        }
        frame #34 {
          # "Get Channel Calibrations"
        }
        frame #35 {
          w568 = u8[] ?  # DATA
          # "Set Channel Calibrations"
          n184 = for {
            N: i32 ? -> [_]
            tunnel: w571 -> [w581]
            shift-right: [w577] -> w569
            shift-left: w568 -> [w578]
            tunnel: [w575] -> w570 mode=indexing
            i -> [w582]
            n185 = Pick Line(multi-line string=w581, line index=w582) -> (output string=w580:string)  [unwired: 1 in]
            n186 = call "Numeric String to Bytes.vi"("Type"=T3 ?, "String"=w580) -> ("error out"=w575:errorcluster, "Byte Data"=w576:u8[])  [unwired: 8 in]
            n187 = Build Array (concatenate)(w578, w576) -> (w577:u8[])
          }
          n188 = Build Array (concatenate)(w570) -> (w567:errorcluster[])
          n189 = call <vilib>:"Merge Errors.vi"("error array in"=w567) -> ("error out"=w572:errorcluster)  [unwired: 6 in]
        }
        frame #36 {
          # "Get Stim ASIC HV Calibrations"
        }
        frame #37 {
          w587 = u8[] ?  # DATA
          # "Set Stim ASIC HV Calibrations"
          n190 = for {
            N: i32 ? -> [_]
            tunnel: w590 -> [w600]
            shift-right: [w596] -> w588
            shift-left: w587 -> [w597]
            tunnel: [w594] -> w589 mode=indexing
            i -> [w601]
            n191 = Pick Line(multi-line string=w600, line index=w601) -> (output string=w599:string)  [unwired: 1 in]
            n192 = call "Numeric String to Bytes.vi"("Type"=T3 ?, "String"=w599) -> ("error out"=w594:errorcluster, "Byte Data"=w595:u8[])  [unwired: 8 in]
            n193 = Build Array (concatenate)(w597, w595) -> (w596:u8[])
          }
          n194 = Build Array (concatenate)(w589) -> (w586:errorcluster[])
          n195 = call <vilib>:"Merge Errors.vi"("error array in"=w586) -> ("error out"=w591:errorcluster)  [unwired: 6 in]
        }
        frame #38 {
          # "Get CP Data"
          n196 = call "Numeric String to Bytes.vi"("Type"=T3 ?, "String"=w607) -> ("error out"=w606:errorcluster, "Byte Data"=w603:u8[])  [unwired: 8 in]
          n197 = Replace Array Subset(array=w608, new element=w603, index=i32 ?) -> (w605:u8[])
        }
        frame #39 {
          # "Set CP Data"
          n198 = Array To Cluster(array=w613) -> (cluster=w611:T5)
          n199 = Pick Line(multi-line string=w617, line index=i32 ?) -> (output string=w619:string)  [unwired: 1 in]
          n200 = Cluster To Array(cluster=w611) -> (array=w612:u8[])
          n201 = call "Numeric String to Bytes.vi"("Type"=T3 ?, "String"=w619) -> ("error out"=w614:errorcluster, "Byte Data"=w615:u8[])  [unwired: 8 in]
          n202 = Build Array (concatenate)(w615, w612) -> (w616:u8[])
          n203 = Build Array(w614) -> (w610:errorcluster[])
          n204 = call <vilib>:"Merge Errors.vi"("error array in"=w610) -> ("error out"=w621:errorcluster)  [unwired: 6 in]
        }
        frame #40 {
          # "Clear Log"
          n205 = call "Numeric String to Bytes.vi"("Type"=T3 ?, "String"=w628) -> ("error out"=w627:errorcluster, "Byte Data"=w624:u8[])  [unwired: 8 in]
          n206 = Replace Array Subset(array=w629, new element=w624, index=i32 ?) -> (w626:u8[])
        }
        frame #41 {
          # "Read Log"
          n207 = Pick Line(multi-line string=w632, line index=i32 ?) -> (output string=w643:string)  [unwired: 1 in]
          n208 = Pick Line(multi-line string=w632, line index=i32 ?) -> (output string=w640:string)  [unwired: 1 in]
          n209 = call "Numeric String to Bytes.vi"("Type"=T3 ?, "String"=w643) -> ("error out"=w636:errorcluster, "Byte Data"=w639:u8[])  [unwired: 8 in]
          n210 = call "Numeric String to Bytes.vi"("Type"=T3 ?, "String"=w640) -> ("error out"=w635:errorcluster, "Byte Data"=w637:u8[])  [unwired: 8 in]
          n211 = Build Array (concatenate)(w639, w637) -> (w638:u8[])
          n212 = Build Array(w636, w635) -> (w634:errorcluster[])
          n213 = Replace Array Subset(array=w648, new element=w638, index=i32 ?) -> (w647:u8[])
          n214 = Build Array (concatenate)(w634) -> (w631:errorcluster[])
          n215 = call <vilib>:"Merge Errors.vi"("error array in"=w631) -> ("error out"=w633:errorcluster)  [unwired: 6 in]
        }
        frame #42 {
          # "Added a U8 Data"
          # "Changed to U16 from U8"
          # "Append Log"
          n216 = Pick Line(multi-line string=w653, line index=i32 ?) -> (output string=w682:string)  [unwired: 1 in]
          n217 = Pick Line(multi-line string=w653, line index=i32 ?) -> (output string=w679:string)  [unwired: 1 in]
          n218 = Pick Line(multi-line string=w653, line index=i32 ?) -> (output string=w669:string)  [unwired: 1 in]
          n219 = Pick Line(multi-line string=w653, line index=i32 ?) -> (output string=w666:string)  [unwired: 1 in]
          n220 = Pick Line(multi-line string=w653, line index=i32 ?) -> (output string=w663:string)  [unwired: 1 in]
          n221 = Pick Line(multi-line string=w653, line index=i32 ?) -> (output string=w656:string)  [unwired: 1 in]
          n222 = call "Numeric String to Bytes.vi"("Type"=T3 ?, "String"=w682) -> ("error out"=w675:errorcluster, "Byte Data"=w678:u8[])  [unwired: 8 in]
          n223 = call "Numeric String to Bytes.vi"("Type"=T3 ?, "String"=w679) -> ("error out"=w674:errorcluster, "Byte Data"=w676:u8[])  [unwired: 8 in]
          n224 = call "Numeric String to Bytes.vi"("Type"=T3 ?, "String"=w669) -> ("error out"=w659:errorcluster, "Byte Data"=w660:u8[])  [unwired: 8 in]
          n225 = call "Numeric String to Bytes.vi"("Type"=T3 ?, "String"=w666) -> ("error out"=w658:errorcluster, "Byte Data"=w661:u8[])  [unwired: 8 in]
          n226 = call "Numeric String to Bytes.vi"("Type"=T3 ?, "String"=w663) -> ("error out"=w657:errorcluster, "Byte Data"=w662:u8[])  [unwired: 8 in]
          n227 = call "Numeric String to Bytes.vi"("Type"=T3 ?, "String"=w656) -> ("error out"=w652:errorcluster, "Byte Data"=w651:u8[])  [unwired: 8 in]
          n228 = Build Array (concatenate)(w678, w676, w660, w661, w662, w651) -> (w677:u8[])
          n229 = Build Array(w675, w674, w659, w658, w657, w652) -> (w673:errorcluster[])
          n230 = Replace Array Subset(array=w687, new element=w677, index=i32 ?) -> (w686:u8[])
          n231 = Build Array (concatenate)(w673) -> (w650:errorcluster[])
          n232 = call <vilib>:"Merge Errors.vi"("error array in"=w650) -> ("error out"=w672:errorcluster)  [unwired: 6 in]
        }
        frame #43 {
          # "Get Patient Program Run-Time"
          n233 = call "Numeric String to Bytes.vi"("Type"=T3 ?, "String"=w694) -> ("error out"=w693:errorcluster, "Byte Data"=w690:u8[])  [unwired: 8 in]
          n234 = Replace Array Subset(array=w695, new element=w690, index=i32 ?) -> (w692:u8[])
        }
        frame #44 {
          # "Set Patient Program Run-Time"
          n235 = Pick Line(multi-line string=w698, line index=i32 ?) -> (output string=w709:string)  [unwired: 1 in]
          n236 = Pick Line(multi-line string=w698, line index=i32 ?) -> (output string=w706:string)  [unwired: 1 in]
          n237 = call "Numeric String to Bytes.vi"("Type"=T3 ?, "String"=w709) -> ("error out"=w702:errorcluster, "Byte Data"=w705:u8[])  [unwired: 8 in]
          n238 = call "Numeric String to Bytes.vi"("Type"=T3 ?, "String"=w706) -> ("error out"=w701:errorcluster, "Byte Data"=w703:u8[])  [unwired: 8 in]
          n239 = Build Array (concatenate)(w705, w703) -> (w704:u8[])
          n240 = Build Array(w702, w701) -> (w700:errorcluster[])
          n241 = Replace Array Subset(array=w714, new element=w704, index=i32 ?) -> (w713:u8[])
          n242 = Build Array (concatenate)(w700) -> (w697:errorcluster[])
          n243 = call <vilib>:"Merge Errors.vi"("error array in"=w697) -> ("error out"=w699:errorcluster)  [unwired: 6 in]
        }
        frame #45 {
          # "Changed to U16 from U8"
          # "Impedance Measurement"
          n244 = Pick Line(multi-line string=w722, line index=i32 ?) -> (output string=w763:string)  [unwired: 1 in]
          n245 = Pick Line(multi-line string=w722, line index=i32 ?) -> (output string=w760:string)  [unwired: 1 in]
          n246 = Pick Line(multi-line string=w722, line index=i32 ?) -> (output string=w750:string)  [unwired: 1 in]
          n247 = Pick Line(multi-line string=w722, line index=i32 ?) -> (output string=w747:string)  [unwired: 1 in]
          n248 = Pick Line(multi-line string=w722, line index=i32 ?) -> (output string=w744:string)  [unwired: 1 in]
          n249 = Pick Line(multi-line string=w722, line index=i32 ?) -> (output string=w735:string)  [unwired: 1 in]
          n250 = Pick Line(multi-line string=w722, line index=i32 ?) -> (output string=w732:string)  [unwired: 1 in]
          n251 = Pick Line(multi-line string=w722, line index=i32 ?) -> (output string=w729:string)  [unwired: 1 in]
          n252 = Pick Line(multi-line string=w722, line index=i32 ?) -> (output string=w723:string)  [unwired: 1 in]
          n253 = call "Numeric String to Bytes.vi"("Type"=T3 ?, "String"=w763) -> ("error out"=w756:errorcluster, "Byte Data"=w759:u8[])  [unwired: 8 in]
          n254 = call "Numeric String to Bytes.vi"("Type"=T3 ?, "String"=w760) -> ("error out"=w755:errorcluster, "Byte Data"=w757:u8[])  [unwired: 8 in]
          n255 = call "Numeric String to Bytes.vi"("Type"=T3 ?, "String"=w750) -> ("error out"=w740:errorcluster, "Byte Data"=w741:u8[])  [unwired: 8 in]
          n256 = call "Numeric String to Bytes.vi"("Type"=T3 ?, "String"=w747) -> ("error out"=w739:errorcluster, "Byte Data"=w742:u8[])  [unwired: 8 in]
          n257 = call "Numeric String to Bytes.vi"("Type"=T3 ?, "String"=w744) -> ("error out"=w738:errorcluster, "Byte Data"=w743:u8[])  [unwired: 8 in]
          n258 = call "Numeric String to Bytes.vi"("Type"=T3 ?, "String"=w735) -> ("error out"=w720:errorcluster, "Byte Data"=w728:u8[])  [unwired: 8 in]
          n259 = call "Numeric String to Bytes.vi"("Type"=T3 ?, "String"=w732) -> ("error out"=w719:errorcluster, "Byte Data"=w727:u8[])  [unwired: 8 in]
          n260 = call "Numeric String to Bytes.vi"("Type"=T3 ?, "String"=w729) -> ("error out"=w718:errorcluster, "Byte Data"=w726:u8[])  [unwired: 8 in]
          n261 = call "Numeric String to Bytes.vi"("Type"=T3 ?, "String"=w723) -> ("error out"=w717:errorcluster, "Byte Data"=w721:u8[])  [unwired: 8 in]
          n262 = Build Array (concatenate)(w759, w757, w741, w742, w743, w728, w727, w726, w721) -> (w758:u8[])
          n263 = Replace Array Subset(array=w768, new element=w758, index=i32 ?) -> (w767:u8[])
          n264 = Build Array(w756, w755, w740, w739, w738, w720, w719, w718, w717) -> (w754:errorcluster[])
          n265 = Build Array (concatenate)(w754) -> (w716:errorcluster[])
          n266 = call <vilib>:"Merge Errors.vi"("error array in"=w716) -> ("error out"=w753:errorcluster)  [unwired: 6 in]
        }
        frame #46 {
          # "Enter Storage Mode"
        }
        frame #47 {
          # "Echo Short"
          n267 = Array Subset(array=w777, index=i32 ?, length=i32 ?) -> (w774:u8[])
        }
        frame #48 {
          # "Echo Long"
          n268 = Array Subset(array=w783, index=i32 ?, length=i32 ?) -> (w780:u8[])
        }
        frame #49 {
          # "Get General Calibration"
        }
        frame #50 {
          w789 = u8[] ?  # DATA
          # "Set General Calibration"
          n269 = disable-structure shown="Disabled" {
            disable-tunnel: [w826 w878] -> w793
            disable-tunnel: [w822 w877] -> w791
            disable-tunnel: w790 -> [w809 w880]
            disable-tunnel: w789 -> [w795 w879]
            frame #0 {
              n270 = for {
                N: i32 ? -> [_]
                tunnel: [w873] -> w827 mode=indexing
                tunnel: w809 -> [w872]
                shift-right: [w869] -> w821
                shift-left: w795 -> [w870]
                tunnel: [w868] -> w805
                i -> [w868]
                n271 = Pick Line(multi-line string=w872, line index=w868) -> (output string=w874:string)  [unwired: 1 in]
                n272 = call "Numeric String to Bytes.vi"("Type"=T3 ?, "String"=w874) -> ("error out"=w873:errorcluster, "Byte Data"=w871:u8[])  [unwired: 8 in]
                n273 = Build Array (concatenate)(w870, w871) -> (w869:u8[])
              }
              n274 = Increment(x=w805) -> (x+1=w804:i32)
              n275 = for {
                N: i32 ? -> [_]
                tunnel: [w835] -> w807 mode=indexing
                tunnel: w809 -> [w834]
                shift-right: [w831] -> w806
                shift-left: w795 -> [w832]
                tunnel: w804 -> [w829]
                tunnel: [w828] -> w802
                i -> [w828]
                n276 = Add(x=w829, y=w828) -> (x+y=w830:i32)
                n277 = Pick Line(multi-line string=w834, line index=w830) -> (output string=w836:string)  [unwired: 1 in]
                n278 = call "Numeric String to Bytes.vi"("Type"=T3 ?, "String"=w836) -> ("error out"=w835:errorcluster, "Byte Data"=w833:u8[])  [unwired: 8 in]
                n279 = Build Array (concatenate)(w832, w833) -> (w831:u8[])
              }
              n280 = Increment(x=w802) -> (x+1=w803:i32)
              n281 = for {
                N: i32 ? -> [_]
                tunnel: [w865] -> w819 mode=indexing
                tunnel: w809 -> [w864]
                shift-right: [w861] -> w820
                shift-left: w795 -> [w862]
                tunnel: w803 -> [w859]
                tunnel: [w858] -> w801
                i -> [w858]
                n282 = Add(x=w859, y=w858) -> (x+y=w860:i32)
                n283 = Pick Line(multi-line string=w864, line index=w860) -> (output string=w866:string)  [unwired: 1 in]
                n284 = call "Numeric String to Bytes.vi"("Type"=T3 ?, "String"=w866) -> ("error out"=w865:errorcluster, "Byte Data"=w863:u8[])  [unwired: 8 in]
                n285 = Build Array (concatenate)(w862, w863) -> (w861:u8[])
              }
              n286 = Increment(x=w801) -> (x+1=w800:i32)
              n287 = for {
                N: i32 ? -> [_]
                tunnel: [w855] -> w816 mode=indexing
                tunnel: w809 -> [w854]
                shift-right: [w851] -> w817
                shift-left: w795 -> [w852]
                tunnel: w800 -> [w849]
                tunnel: [w848] -> w798
                i -> [w848]
                n288 = Add(x=w849, y=w848) -> (x+y=w850:i32)
                n289 = Pick Line(multi-line string=w854, line index=w850) -> (output string=w856:string)  [unwired: 1 in]
                n290 = call "Numeric String to Bytes.vi"("Type"=T3 ?, "String"=w856) -> ("error out"=w855:errorcluster, "Byte Data"=w853:u8[])  [unwired: 8 in]
                n291 = Build Array (concatenate)(w852, w853) -> (w851:u8[])
              }
              n292 = Increment(x=w798) -> (x+1=w799:i32)
              n293 = for {
                N: i32 ? -> [_]
                tunnel: [w845] -> w813 mode=indexing
                tunnel: w809 -> [w844]
                shift-right: [w841] -> w814
                shift-left: _ -> [w842]
                tunnel: w799 -> [w839]
                tunnel: [w838] -> w797
                i -> [w838]
                n294 = Add(x=w839, y=w838) -> (x+y=w840:i32)
                n295 = Pick Line(multi-line string=w844, line index=w840) -> (output string=w846:string)  [unwired: 1 in]
                n296 = call "Numeric String to Bytes.vi"("Type"=T3 ?, "String"=w846) -> ("error out"=w845:errorcluster, "Byte Data"=w843:u8[])  [unwired: 8 in]
                n297 = Build Array (concatenate)(w842, w843) -> (w841:u8[])
              }
              n298 = Increment(x=w797) -> (x+1=w796:i32)
              n299 = Pick Line(multi-line string=w809, line index=w796) -> (output string=w824:string)  [unwired: 1 in]
              n300 = call "Numeric String to Bytes.vi"("Type"=T3 ?, "String"=w824) -> ("error out"=w812:errorcluster, "Byte Data"=w811:u8[])  [unwired: 8 in]
              n301 = Build Array (concatenate)(w821, w806, w820, w817, w814, w811) -> (w822:u8[])
              n302 = Build Array (concatenate)(w827, w807, w819, w816, w813, w812) -> (w826:errorcluster[])
            }
            frame #1 {
              n303 = for {
                N: i32 ? -> [_]
                tunnel: [w886] -> w878 mode=indexing
                tunnel: w880 -> [w885]
                shift-right: [w882] -> w877
                shift-left: w879 -> [w883]
                i -> [w881]
                n304 = Pick Line(multi-line string=w885, line index=w881) -> (output string=w887:string)  [unwired: 1 in]
                n305 = call "Numeric String to Bytes.vi"("Type"=T3 ?, "String"=w887) -> ("error out"=w886:errorcluster, "Byte Data"=w884:u8[])  [unwired: 8 in]
                n306 = Build Array (concatenate)(w883, w884) -> (w882:u8[])
              }
            }
          }
          n307 = Build Array (concatenate)(w793) -> (w788:errorcluster[])
          n308 = call <vilib>:"Merge Errors.vi"("error array in"=w788) -> ("error out"=w792:errorcluster)  [unwired: 6 in]
        }
        frame #51 {
          # "Changed to U8 from U16"
          # "Get Trim List"
          n309 = call "Numeric String to Bytes.vi"("Type"=T3 ?, "String"=w891) -> ("error out"=w890:errorcluster, "Byte Data"=w894:u8[])  [unwired: 8 in]
          n310 = Replace Array Subset(array=w892, new element=w894, index=i32 ?) -> (w889:u8[])
        }
        frame #52 {
          w916 = u8[] ?  # DATA
          # "Set Trim List"
          n311 = Pick Line(multi-line string=w906, line index=i32 ?) -> (output string=w915:string)  [unwired: 1 in]
          n312 = Pick Line(multi-line string=w906, line index=i32 ?) -> (output string=w911:string)  [unwired: 1 in]
          n313 = call "Numeric String to Bytes.vi"("Type"=T3 ?, "String"=w915) -> ("error out"=w900:errorcluster, "Byte Data"=w912:u8[])  [unwired: 8 in]
          n314 = call "Numeric String to Bytes.vi"("Type"=T3 ?, "String"=w911) -> ("error out"=w899:errorcluster, "Byte Data"=w909:u8[])  [unwired: 8 in]
          n315 = Index Array(array=w909, index=i32 ?) -> (element=w908:u8)
          n316 = for {
            N: w908 -> [_]
            tunnel: w906 -> [w919]
            shift-right: [w932] -> w898
            shift-left: w916 -> [w933]
            tunnel: [w930] -> w903 mode=indexing
            tunnel: [w927] -> w901 mode=indexing
            i -> [w921]
            w922 = i32 ? ("y")
            n317 = Multiply(x=w922, y=w921) -> (x*y=w923:i32)
            n318 = Add(x=w922, y=w923) -> (x+y=w926:i32)
            n319 = Add(x=w923, y=i32 ?) -> (x+y=w925:i32)
            n320 = Pick Line(multi-line string=w919, line index=w926) -> (output string=w935:string)  [unwired: 1 in]
            n321 = Pick Line(multi-line string=w919, line index=w925) -> (output string=w929:string)  [unwired: 1 in]
            n322 = call "Numeric String to Bytes.vi"("Type"=T3 ?, "String"=w935) -> ("error out"=w930:errorcluster, "Byte Data"=w931:u8[])  [unwired: 8 in]
            n323 = call "Numeric String to Bytes.vi"("Type"=T3 ?, "String"=w929) -> ("error out"=w927:errorcluster, "Byte Data"=w920:u8[])  [unwired: 8 in]
            n324 = Build Array (concatenate)(w933, w931, w920) -> (w932:u8[])
          }
          n325 = Build Array (concatenate)(w912, w909, w898) -> (w913:u8[])
          n326 = Build Array (concatenate)(w903, w901, w900, w899) -> (w902:errorcluster[])
          n327 = Build Array (concatenate)(w902) -> (w897:errorcluster[])
          n328 = call <vilib>:"Merge Errors.vi"("error array in"=w897) -> ("error out"=w917:errorcluster)  [unwired: 6 in]
        }
        frame #53 {
          # "Get Counter"
          n329 = call "Numeric String to Bytes.vi"("Type"=T3 ?, "String"=w941) -> ("error out"=w940:errorcluster, "Byte Data"=w937:u8[])  [unwired: 8 in]
          n330 = Replace Array Subset(array=w942, new element=w937, index=i32 ?) -> (w939:u8[])
        }
        frame #54 {
          # "Set Counter"
          n331 = Pick Line(multi-line string=w945, line index=i32 ?) -> (output string=w956:string)  [unwired: 1 in]
          n332 = Pick Line(multi-line string=w945, line index=i32 ?) -> (output string=w953:string)  [unwired: 1 in]
          n333 = call "Numeric String to Bytes.vi"("Type"=T3 ?, "String"=w956) -> ("error out"=w949:errorcluster, "Byte Data"=w952:u8[])  [unwired: 8 in]
          n334 = call "Numeric String to Bytes.vi"("Type"=T3 ?, "String"=w953) -> ("error out"=w948:errorcluster, "Byte Data"=w950:u8[])  [unwired: 8 in]
          n335 = Build Array (concatenate)(w952, w950) -> (w951:u8[])
          n336 = Build Array(w949, w948) -> (w947:errorcluster[])
          n337 = Replace Array Subset(array=w961, new element=w951, index=i32 ?) -> (w960:u8[])
          n338 = Build Array (concatenate)(w947) -> (w944:errorcluster[])
          n339 = call <vilib>:"Merge Errors.vi"("error array in"=w944) -> ("error out"=w946:errorcluster)  [unwired: 6 in]
        }
        frame #55 {
          # "Get Test Stimulation"
        }
        frame #56 {
          w983 = u8[] ?  # DATA
          # "Set Test Stimulation"
          n340 = for {
            N: i32 ? -> [_]
            shift-right: [w1029] -> w968
            shift-left: w983 -> [w1031]
            tunnel: w971 -> [w1008]
            shift-right: [w1004] -> _
            shift-left: i32 ? ("line index") -> [w1034]
            tunnel: [w1026] -> w988 mode=indexing
            w1027 = u8[] ?  # DATA
            n341 = Increment(x=w1034) -> (x+1=w1025:i32)
            n342 = Pick Line(multi-line string=w1008, line index=w1034) -> (output string=w1032:string)  [unwired: 1 in]
            n343 = for {
              N: i32 ? -> [_]
              tunnel: w1008 -> [w1043]
              shift-right: [w1038] -> w1006
              shift-left: w1027 -> [w1039]
              shift-right: [w1036] -> w1016
              shift-left: w1025 -> [w1037]
              tunnel: [w1035] -> _ mode=indexing
              n344 = Pick Line(multi-line string=w1043, line index=w1037) -> (output string=w1041:string)  [unwired: 1 in]
              n345 = Increment(x=w1037) -> (x+1=w1036:i32)
              n346 = call "Numeric String to Bytes.vi"("Type"=T3 ?, "String"=w1041) -> ("error out"=w1035:errorcluster, "Byte Data"=w1040:u8[])  [unwired: 8 in]
              n347 = Build Array (concatenate)(w1039, w1040) -> (w1038:u8[])
            }
            n348 = Increment(x=w1016) -> (x+1=w1015:i32)
            n349 = Pick Line(multi-line string=w1008, line index=w1016) -> (output string=w1024:string)  [unwired: 1 in]
            n350 = Increment(x=w1015) -> (x+1=w1014:i32)
            n351 = Pick Line(multi-line string=w1008, line index=w1015) -> (output string=w1021:string)  [unwired: 1 in]
            n352 = Increment(x=w1014) -> (x+1=w1012:i32)
            n353 = Pick Line(multi-line string=w1008, line index=w1014) -> (output string=w1019:string)  [unwired: 1 in]
            n354 = Increment(x=w1012) -> (x+1=w1007:i32)
            n355 = Pick Line(multi-line string=w1008, line index=w1012) -> (output string=w1018:string)  [unwired: 1 in]
            n356 = call "Numeric String to Bytes.vi"("Type"=T3 ?, "String"=w1032) -> ("error out"=w997:errorcluster, "Byte Data"=w1030:u8[])  [unwired: 8 in]
            n357 = Increment(x=w1007) -> (x+1=w1005:i32)
            n358 = Pick Line(multi-line string=w1008, line index=w1007) -> (output string=w1017:string)  [unwired: 1 in]
            n359 = Pick Line(multi-line string=w1008, line index=w1005) -> (output string=w1009:string)  [unwired: 1 in]
            n360 = call "Numeric String to Bytes.vi"("Type"=T3 ?, "String"=w1024) -> ("error out"=w996:errorcluster, "Byte Data"=w1003:u8[])  [unwired: 8 in]
            n361 = call "Numeric String to Bytes.vi"("Type"=T3 ?, "String"=w1021) -> ("error out"=w995:errorcluster, "Byte Data"=w1002:u8[])  [unwired: 8 in]
            n362 = call "Numeric String to Bytes.vi"("Type"=T3 ?, "String"=w1019) -> ("error out"=w994:errorcluster, "Byte Data"=w1001:u8[])  [unwired: 8 in]
            n363 = call "Numeric String to Bytes.vi"("Type"=T3 ?, "String"=w1018) -> ("error out"=w993:errorcluster, "Byte Data"=w1000:u8[])  [unwired: 8 in]
            n364 = call "Numeric String to Bytes.vi"("Type"=T3 ?, "String"=w1017) -> ("error out"=w992:errorcluster, "Byte Data"=w999:u8[])  [unwired: 8 in]
            n365 = call "Numeric String to Bytes.vi"("Type"=T3 ?, "String"=w1009) -> ("error out"=w991:errorcluster, "Byte Data"=w998:u8[])  [unwired: 8 in]
            n366 = Build Array (concatenate)(w1031, w1030, w1006, w1003, w1002, w1001, w1000, w999, w998) -> (w1029:u8[])
            n367 = Build Array(w997, w996, w995, w994, w993, w992, w991) -> (w990:errorcluster[])
            n368 = call <vilib>:"Merge Errors.vi"("error array in"=w990) -> ("error out"=w1026:errorcluster)  [unwired: 6 in]
            n369 = Increment(x=w1005) -> (x+1=w1004:i32)
          }
          n370 = Pick Line(multi-line string=w971, line index=i32 ?) -> (output string=w972:string)  [unwired: 1 in]
          n371 = Pick Line(multi-line string=w971, line index=i32 ?) -> (output string=w978:string)  [unwired: 1 in]
          n372 = Pick Line(multi-line string=w971, line index=i32 ?) -> (output string=w981:string)  [unwired: 1 in]
          n373 = call "Numeric String to Bytes.vi"("Type"=T3 ?, "String"=w972) -> ("Byte Data"=w970:u8[])  [unwired: 8 in, 1 out]
          n374 = call "Numeric String to Bytes.vi"("Type"=T3 ?, "String"=w978) -> ("error out"=w986:errorcluster, "Byte Data"=w975:u8[])  [unwired: 8 in]
          n375 = call "Numeric String to Bytes.vi"("Type"=T3 ?, "String"=w981) -> ("error out"=w987:errorcluster, "Byte Data"=w985:u8[])  [unwired: 8 in]
          n376 = Build Array (concatenate)(w975, w985, w970, w968) -> (w967:u8[])
          n377 = Build Array (concatenate)(w986, w987, w988) -> (w966:errorcluster[])
          n378 = call <vilib>:"Merge Errors.vi"("error array in"=w966) -> ("error out"=w969:errorcluster)  [unwired: 6 in]
        }
        frame #57 {
          # "Get Titration Stimulation"
        }
        frame #58 {
          w1058 = u8[] ?  # DATA
          # "Set Titration Stimulation"
          n379 = for {
            N: i32 ? -> [_]
            shift-right: [w1079] -> w1053
            shift-left: w1058 -> [w1082]
            tunnel: w1057 -> [w1068]
            shift-right: [w1073] -> _
            shift-left: i32 ? ("line index") -> [w1087]
            tunnel: [w1069] -> w1049 mode=indexing
            w1075 = u8[] ?  # DATA
            n380 = Increment(x=w1087) -> (x+1=w1077:i32)
            n381 = Pick Line(multi-line string=w1068, line index=w1087) -> (output string=w1084:string)  [unwired: 1 in]
            n382 = Pick Line(multi-line string=w1068, line index=w1077) -> (output string=w1083:string)  [unwired: 1 in]
            n383 = Increment(x=w1077) -> (x+1=w1076:i32)
            n384 = call "Numeric String to Bytes.vi"("Type"=T3 ?, "String"=w1084) -> ("error out"=w1072:errorcluster, "Byte Data"=w1081:u8[])  [unwired: 8 in]
            n385 = call "Numeric String to Bytes.vi"("Type"=T3 ?, "String"=w1083) -> ("error out"=w1071:errorcluster, "Byte Data"=w1080:u8[])  [unwired: 8 in]
            n386 = for {
              N: i32 ? -> [_]
              tunnel: w1068 -> [w1096]
              shift-right: [w1091] -> w1074
              shift-left: w1075 -> [w1092]
              shift-right: [w1089] -> w1073
              shift-left: w1076 -> [w1090]
              tunnel: [w1088] -> w1070 mode=indexing
              n387 = Pick Line(multi-line string=w1096, line index=w1090) -> (output string=w1094:string)  [unwired: 1 in]
              n388 = Increment(x=w1090) -> (x+1=w1089:i32)
              n389 = call "Numeric String to Bytes.vi"("Type"=T3 ?, "String"=w1094) -> ("error out"=w1088:errorcluster, "Byte Data"=w1093:u8[])  [unwired: 8 in]
              n390 = Build Array (concatenate)(w1092, w1093) -> (w1091:u8[])
            }
            n391 = Build Array (concatenate)(w1082, w1081, w1080, w1074) -> (w1079:u8[])
            n392 = Build Array (concatenate)(w1072, w1071, w1070) -> (w1067:errorcluster[])
            n393 = call <vilib>:"Merge Errors.vi"("error array in"=w1067) -> ("error out"=w1069:errorcluster)  [unwired: 6 in]
          }
          n394 = Pick Line(multi-line string=w1057, line index=i32 ?) -> (output string=w1063:string)  [unwired: 1 in]
          n395 = Pick Line(multi-line string=w1057, line index=i32 ?) -> (output string=w1060:string)  [unwired: 1 in]
          n396 = call "Numeric String to Bytes.vi"("Type"=T3 ?, "String"=w1063) -> ("error out"=w1051:errorcluster, "Byte Data"=w1055:u8[])  [unwired: 8 in]
          n397 = call "Numeric String to Bytes.vi"("Type"=T3 ?, "String"=w1060) -> ("error out"=w1050:errorcluster, "Byte Data"=w1054:u8[])  [unwired: 8 in]
          n398 = Build Array (concatenate)(w1055, w1054, w1053) -> (w1052:u8[])
          n399 = Build Array (concatenate)(w1051, w1050, w1049) -> (w1047:errorcluster[])
          n400 = call <vilib>:"Merge Errors.vi"("error array in"=w1047) -> ("error out"=w1048:errorcluster)  [unwired: 6 in]
        }
        frame #59 {
          # "Get Ramp Time"
        }
        frame #60 {
          # "Set Ramp Time"
          n401 = call "Numeric String to Bytes.vi"("Type"=T3 ?, "String"=w1104) -> ("error out"=w1100:errorcluster, "Byte Data"=w1102:u8[])  [unwired: 8 in]
          n402 = Replace Array Subset(array=w1103, new element=w1102, index=i32 ?) -> (w1101:u8[])
        }
        frame #61 {
          # "Get VBAT"
        }
        frame #62 {
          # "Set Software Description Block"
        }
        frame #63 {
          # "Get Software Description Block"
        }
        frame #64 {
          # "Write Memory"
          n403 = Array Subset(array=w1119, index=i32 ?, length=i32 ?) -> (w1118:u8[])
          n404 = Pick Line(multi-line string=w1124, line index=i32 ?) -> (output string=w1132:string)  [unwired: 1 in]
          n405 = Pick Line(multi-line string=w1124, line index=i32 ?) -> (output string=w1129:string)  [unwired: 1 in]
          n406 = call "Numeric String to Bytes.vi"("Type"=T3 ?, "String"=w1132) -> ("error out"=w1126:errorcluster, "Byte Data"=w1128:u8[])  [unwired: 8 in]
          n407 = call "Numeric String to Bytes.vi"("Type"=T3 ?, "String"=w1129) -> ("error out"=w1125:errorcluster, "Byte Data"=w1127:u8[])  [unwired: 8 in]
          n408 = Build Array (concatenate)(w1128, w1127, w1118) -> (w1123:u8[])
          n409 = Build Array(w1126, w1125) -> (w1117:errorcluster[])
          n410 = call <vilib>:"Merge Errors.vi"("error array in"=w1117) -> ("error out"=w1122:errorcluster)  [unwired: 6 in]
        }
        frame #65 {
          # "Read Memory"
          n411 = Pick Line(multi-line string=w1148, line index=i32 ?) -> (output string=w1150:string)  [unwired: 1 in]
          n412 = Pick Line(multi-line string=w1148, line index=i32 ?) -> (output string=w1146:string)  [unwired: 1 in]
          n413 = call "Numeric String to Bytes.vi"("Type"=T3 ?, "String"=w1150) -> ("error out"=w1141:errorcluster, "Byte Data"=w1143:u8[])  [unwired: 8 in]
          n414 = call "Numeric String to Bytes.vi"("Type"=T3 ?, "String"=w1146) -> ("error out"=w1140:errorcluster, "Byte Data"=w1142:u8[])  [unwired: 8 in]
          n415 = Build Array (concatenate)(w1143, w1142) -> (w1144:u8[])
          n416 = Build Array(w1141, w1140) -> (w1136:errorcluster[])
          n417 = call <vilib>:"Merge Errors.vi"("error array in"=w1136) -> ("error out"=w1139:errorcluster)  [unwired: 6 in]
          n418 = Replace Array Subset(array=w1138, new element=w1144, index=i32 ?) -> (w1137:u8[])
        }
        frame #66 {
          # "Reset xPG"
        }
        frame #67 {
          # "Erase Flash Block"
        }
        frame #68 {
          # "Write Vectors"
        }
        frame #69 {
          # "Read Vectors"
        }
        frame #70 {
          # "Diagnostic  Data"
          n419 = Pick Line(multi-line string=w1179, line index=i32 ?) -> (output string=w1180:string)  [unwired: 1 in]
          n420 = Pick Line(multi-line string=w1179, line index=i32 ?) -> (output string=w1176:string)  [unwired: 1 in]
          n421 = call "Numeric String to Bytes.vi"("Type"=T3 ?, "String"=w1180) -> ("error out"=w1173:errorcluster, "Byte Data"=w1175:u8[])  [unwired: 8 in]
          n422 = call "Numeric String to Bytes.vi"("Type"=T3 ?, "String"=w1176) -> ("error out"=w1172:errorcluster, "Byte Data"=w1174:u8[])  [unwired: 8 in]
          n423 = Build Array (concatenate)(w1175, w1174) -> (w1168:u8[])
          n424 = Build Array(w1173, w1172) -> (w1166:errorcluster[])
          n425 = call <vilib>:"Merge Errors.vi"("error array in"=w1166) -> ("error out"=w1171:errorcluster)  [unwired: 6 in]
          n426 = Replace Array Subset(array=w1170, new element=w1168, index=i32 ?) -> (w1167:u8[])
        }
        frame #71 {
          # "Set Background Impedance"
          n427 = Pick Line(multi-line string=w1191, line index=i32 ?) -> (output string=w1197:string)  [unwired: 1 in]
          n428 = Pick Line(multi-line string=w1191, line index=i32 ?) -> (output string=w1195:string)  [unwired: 1 in]
          n429 = Pick Line(multi-line string=w1191, line index=i32 ?) -> (output string=w1193:string)  [unwired: 1 in]
          n430 = Pick Line(multi-line string=w1191, line index=i32 ?) -> (output string=w1190:string)  [unwired: 1 in]
          n431 = call "Numeric String to Bytes.vi"("Type"=T3 ?, "String"=w1197) -> ("error out"=w1189:errorcluster, "Byte Data"=w1206:u8[])  [unwired: 8 in]
          n432 = call "Numeric String to Bytes.vi"("Type"=T3 ?, "String"=w1195) -> ("error out"=w1188:errorcluster, "Byte Data"=w1204:u8[])  [unwired: 8 in]
          n433 = call "Numeric String to Bytes.vi"("Type"=T3 ?, "String"=w1193) -> ("error out"=w1187:errorcluster, "Byte Data"=w1202:u8[])  [unwired: 8 in]
          n434 = call "Numeric String to Bytes.vi"("Type"=T3 ?, "String"=w1190) -> ("error out"=w1186:errorcluster, "Byte Data"=w1200:u8[])  [unwired: 8 in]
          n435 = Build Array (concatenate)(w1206, w1204, w1202, w1200) -> (w1199:u8[])
          n436 = Build Array(w1189, w1188, w1187, w1186) -> (w1184:errorcluster[])
          n437 = call <vilib>:"Merge Errors.vi"("error array in"=w1184) -> ("error out"=w1185:errorcluster)  [unwired: 6 in]
        }
        frame #72 {
          # "Get Background Impedance"
        }
      }
      n438 = Increment(x=w15) -> (x+1=w3:T1)
      n439 = while {
        tunnel: w3 -> [w20]
        tunnel: "EXID" -> [w19]
        shift-right: [w21] -> _
        shift-left: w13 -> [w22]
        tunnel: w10 -> [w17]
        tunnel: [w16] -> w12 mode=indexing
        i -> [w23]
        stop <- w18 continue-if-true
        n440 = case shown="1, Default" w23 {
          tunnel: w22 -> [w46 w56]
          tunnel: [w45 w60] -> w21
          tunnel: w20 -> [w26 _]
          tunnel: w19 -> [w42 _]
          tunnel: [w43 w58] -> w18
          tunnel: w17 -> [w38 w50]
          tunnel: [w29 w52] -> w16
          frame #0 {
            n441 = Split Number(x=w42) -> (hi(x)=w41:u16, lo(x)=w40:u16)
            n442 = Array To Cluster(array=w38) -> (cluster=w39:T6)
            n443 = Split Number(x=w41) -> (lo(x)=w36:u8)  [unwired: 1 out]
            n444 = Split Number(x=w40) -> (hi(x)=w37:u8, lo(x)=w35:u8)
            n445 = Delete From Array(array=w46, length=i32 ?, index=i32 ?) -> (deleted portion=w31:u8[], array with subset deleted=w45:u8[])
            n446 = Split Number(x=w26) -> (hi(x)=w27:u8, lo(x)=w28:u8)
            n447 = Bundle By Name(cluster=w39, "DATA[5]"=w27, "DATA[4]"=w28, "DATA[3]"=w36, "DATA[2]"=w37, "DATA[1]"=w35, "DATA[0]"=i32 ?) -> (w33:T6)
            n448 = Cluster To Array(cluster=w33) -> (array=w30:u8[])
            n449 = Array Size(array=w45) -> (size(s)=w44:i32)
            n450 = Replace Array Subset(array=w30, new element=w31, index=i32 ?) -> (w29:u8[])
            n451 = Greater Than 0?(x=w44) -> (x > 0?=w43:bool)
          }
          frame #1 {
            n452 = Delete From Array(array=w56, length=i32 ? ("index"), index=i32 ? ("length")) -> (deleted portion=w49:u8[], array with subset deleted=w60:u8[])
            n453 = Array Size(array=w56) -> (size(s)=w55:i32)
            n454 = Array Size(array=w60) -> (size(s)=w59:i32)
            n455 = Replace Array Subset(array=w50, new element=w49, index=i32 ?) -> (w52:u8[])
            n456 = Greater?(x=w55, y=i32 ? ("index")) -> (0:w54:bool)
            n457 = Greater Than 0?(x=w59) -> (x > 0?=w57:bool)
            n458 = Or(x=w54, y=w57) -> (x .or. y?=w58:bool)
          }
        }
      }
      n459 = Transpose 2D Array(2D array=w12) -> (transposed array=→"Downlink":u8[][])
    }
    frame #1 {
    }
  }
  "error out" <- w2
  n460 = disable-structure shown="Enabled" {
    frame #0 {
    }
    frame #1 {
    }
  }
